vi "AlliGator Phasor Calibration Actions.vi"(0 "AlliGator Q Elements":T6[](array[typedef]), 1 "VI in":refnum<vi>, 2 "Script in":bool, 5 "data value reference":refnum<data-value>, 7 "AlliGator Q Event in":T7=enum."GUI:Idle", 9 "Data":variant, 11 "error in (no error)":errorcluster, 12 "AlliGator Ctrl Refnums":T8) -> (3 "Script out":bool, 4 "Alligator Queue Element 1 (+ 2)":T6[](array[typedef]), 6 "AlliGator IV DVR":refnum<data-value>, 10 "[Notebook Message]":T1[](array[typedef]) {"Message Style"."Font Size" min=6.0 step=1.0}, 15 "error out":errorcluster)   [LabVIEW 2021, in "AlliGator Action Engine.lvlib"]
doc: "Processes AlliGator phasor calibration-related actions."
uses:
  AlliGator Action Engine.lvlib
  Internal Variables/AlliGator Internal Variables v2.ctl
  <vilib>/vision/Image Controls.llb/IMAQ Image.ctl
  Internal Variables/AlliGator Gate Image Set.ctl
  Files/AlliGator FLI Dataset Type.ctl
  Files/AlliGator Data Series Type.ctl
  Dual-Channel Datasets/AlliGator Dataset Channel.ctl
  Settings/AlliGator Gate Arithmetic.ctl
  Source Image/AlliGator Displayed Image.ctl
  Image/Named ROI Description.ctl
  Phasor Graph/AlliGator Decay Metadata v3.ctl
  Decay Analysis/Decay Preprocessing/AlliGator Decay Background Subtraction Info.ctl
  Decay Analysis/Decay Preprocessing/AlliGator Baseline Subtraction Method.ctl
  Graphs/XY Graph/XY Graph Plot Shift Parameters.ctl
  Graphs/XY Graph/XY Graph Plot Shift Method.ctl
  Decay Analysis/Decay Preprocessing/AlliGator Decay Extrapolation Parameters.ctl
  Phasor/Calibration Phasor (m, phi).ctl
  Phasor/Phasor Reference Series.ctl
  Phasor/Phasor Calibration Map v2.ctl
  Phasor/Phasor (g, s).ctl
  Phasor Graph/AlliGator Raw Phasor Plot Data v5.ctl
  Phasor/Phasor Standard Deviation Options.ctl
  Phasor Plot/AlliGator Phasor Multi-Harmonic Data.ctl
  Phasor/Phasor Harmonic Data.ctl
  Decay Fit Parameter Map/AlliGator Decay Fit Options & Parameters v4.ctl
  Fits/IRF(X)PSED/Decay Fit Options v4.ctl
  Fits/Decay Convolution/Decay Model.ctl
  Fits/Residual Type.ctl
  Fits/IRF(X)PSED/Fit Weights Type v2.ctl
  Fits/Non-linear Fitting Method v2.ctl
  Fits/Fit Calculation Method.ctl
  Fits/Non-linear Fitting Algorithm.ctl
  Decay Analysis/Decay Fit/AlliGator Decay Fit Parameter Constraints 2.ctl
  Fits/IRF(X)PSED/Decay Fit Parameters In List.ctl
  Fits/IRF(X)PSED/MLE Baseline Offset Type.ctl
  Decay Analysis/Decay Preprocessing/AlliGator Decay Preprocessing Parameters.ctl
  Fits/IRF(X)PSED/Decay Fit Parameters & Derived Quantities List v2.ctl
  Fits/IRF(X)PSED/Decay Fit Result Constraint.ctl
  Decay Fit Parameter Map/AlliGator Parameter Maps Data.ctl
  AlliGator Q Event.ctl
  GUI/AlliGator Ctrl Refnums.ctl
  GUI/AlliGator Other Ctrl Refnums.ctl
  GUI/AlliGator State Indicator.ctl
  GUI/AlliGator Main Window Tabs.ctl
  GUI/AlliGator Phasor Plot Ctrl Refnums.ctl
  GUI/AlliGator Phasor Graph Ctrl Refnums.ctl
  Phasor/Phasor Calibration Type.ctl
  GUI/AlliGator Dataset Ctrl Refnums.ctl
  GUI/AlliGator Registered Events Ctrl Refnums.ctl
  GUI/AlliGator Image Histogram Control Refnums.ctl
  Histograms/Linear Histogram Options.ctl
  Histograms/Histogram Bin Option.ctl
  Histograms/Histogram Bin Position.ctl
  Decay Fit Parameter Map/AlliGator Decay Fit Map Control Refnums.ctl
  Parameter Map/AlliGator Parameter Map Control Refnums.ctl
  AlliGator Q Element.ctl
  Notebook/Notebook Message Object.ctl
  Rich Text Box/Text Formatting.ctl
  Rich Text Box/Text Colors.ctl
  Rich Text Box/Text Style.ctl
  Rich Text Box/Text Alignment.ctl
  Alligator Elements Order in Action Stack.ctl
  AlliGator State Indicators List.ctl
  Rich Text Box/Text Format List.ctl
  Graphs/XY Graph/XY Graph Mouse Click Event Data.ctl
  Graphs/XY Graph/XY Graph Refnum.ctl
  <vilib>/Utility/miscctls.llb/LVPoint32TypeDef.ctl
  Files/Load-Save File Info.ctl
  Variant/Variant to Data/Variant to I32.vi
  Variant/Variant to Data/Variant to Boolean.vi
  AlliGator Add Single Action to Stack.vi
  Graphs/Get Plot at Mouse Click (XY Graph)/Get Plot at Mouse Click [AAC].vi
  AlliGator Add Action Array to Stack.vi
  Phasor/Phasor.lvlib
  Settings/AlliGator Settings.lvlib
  Phasor Calibration/AlliGator Phasor Calibration.lvlib
  Files/Files.lvlib
  GUI/AlliGator GUI.lvlib
  Graphs/XY Graph/XY Graph Add-Ons.lvlib
  Graphs/Graphs.lvlib
  GUI/GUI.lvlib
  Phasor Graph/AlliGator Phasor Graph.lvlib
  Variant/Variant to Data/Variant to Data.lvlib
  Internal Variables/AlliGator Internal Variables.lvlib
  Sound/Sound.lvlib
  Notebook/Notebook.lvlib
  Source Image/AlliGator Source Image.lvlib
  Decay Fit Parameter Map/AlliGator Decay Fit Parameter Map.lvlib
  Image/Image.lvlib
  Decay Analysis/Decay Preprocessing/AlliGator Decay Preprocessing.lvlib
  Files/AlliGator Files.lvlib
  Phasor Plot/AlliGator Phasor Plot.lvlib
  Fits/Fits.lvlib
  Decay Analysis/Decay Fit/AlliGator Decay Fit.lvlib
  Rich Text Box/Rich Text Box.lvlib
  Dual-Channel Datasets/AlliGator Dual-Channel Datasets.lvlib
  Histograms/Histogram Window.lvlib
  Parameter Map/AlliGator Parameter Map.lvlib
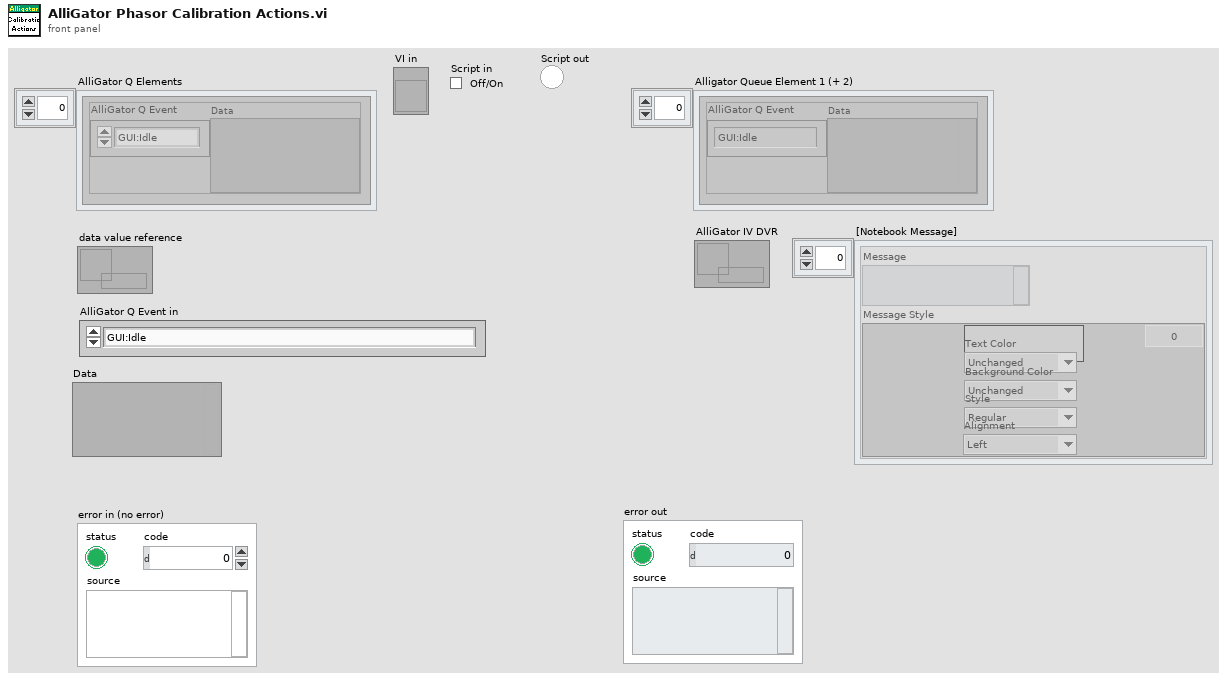
[diagram p1: front panel]
types:
  T1 = typedef "Notebook.lvlib/Notebook Message Object.ctl" = cluster{"Message":string, "Message Style":T2}
  T2 = typedef "Rich Text Box.lvlib/Text Formatting.ctl" = cluster{"Font":string, "Text Color":T3, "Background Color":T3, "Style":T4, "Font Size":dbl, "Alignment":T5}
  T3 = typedef "Rich Text Box.lvlib/Text Colors.ctl" = enum16{"Unchanged", "Black", "Blue", "Cyan", "Maroon", "Gray", "Violet", "Green", "Light Green", "Orange", "Yellow", "Magenta", "Red", "White"}
  T4 = typedef "Rich Text Box.lvlib/Text Style.ctl" = enum16{"Regular", "Bold", "Italic", "Underline", "Strikeout"}
  T5 = typedef "Rich Text Box.lvlib/Text Alignment.ctl" = enum16{"Left", "Right", "Center"}
  T6 = typedef "AlliGator Action Engine.lvlib/AlliGator Q Element.ctl" = cluster{"AlliGator Q Event":T7, "Data":variant}
  T7 = typedef "AlliGator Action Engine.lvlib/AlliGator Q Event.ctl" = enum16{"---- Files ----", "Files:Set Batch Export Files To Save", "Files:Set Dataset Loading & Pre-processing Options", "Files:Check #Frames in Dataset", "Files:Increment Frame Index", "Files:Open Mask Image", "Files:Open White Light Image", "Files:Open Single Dataset", "Files:New Folder of Folders Selected", "Files:Load File (all Types)_Scriptable", "Files:Move Flattened Series to Folders Series", "Files:Select Folder", "Files:Load FLI Dataset", "Files:Load Swiss SPAD 1 Dataset", "Files:Load Swiss SPAD 2 Dataset", "Files:Load .sdt FLI Dataset", "Files:Load .ptu FLI Dataset", "Files:Load .bin FLI Dataset", "Files:Load Single Gate Image Folder", "Files:Load I/m/phi Dataset (deprecated)", "Files:Load Single Image", "Files:Subtract Background File", "Files:Export FLI Dataset", "Files:Load HDF5 FLI Dataset", "Files:Set Destination File Path", "Files:Save Mask Image", "Files:Batch Conversion", "Files:New Folder Selected", "Files:Close FLI Dataset", "Files:Close FLI Dataset Series", "Files:Close White Light Image", "Files:Close Mask Image", "---- FLI Dataset ----", "FLI Dataset:Channel Arithmetic", "FLI Dataset:Export Average Lifetime Map as ASCII", "FLI Dataset:Export User-Defined Quantity Map as ASCII", "FLI Dataset:Python Function FLI Dataset Event", "FLI Dataset:ROI Analysis", "FLI Dataset:Tilted Logistic Square Gated IRF Characteristics Map", "FLI Dataset:Logistic Square Gated IRF Characteristics Map", "FLI Dataset:Square Gated IRF Characteristics Map", "FLI Dataset:Multi-ROI Single-Pixel Phasor Analysis", "FLI Dataset:Multi-ROI Single-Pixel NLSF Analysis", "FLI Dataset:All ROIs IRF Extraction", "FLI Dataset:All ROIs Decay Fit Non-Interactive (Fast + Individual IRF)", "FLI Dataset:All ROIs Phasor Analysis", "FLI Dataset:All ROIs Decay Fit", "FLI Dataset:Fluorescence Decay Statistics", "FLI Dataset:Update Decay Statistics Graph", "FLI Dataset:Get Decay from ROI", "FLI Dataset:All ROIs Average Lifetimes", "FLI Dataset:Save/Load Local IRFs", "FLI Dataset:Clear Local IRFs", "FLI Dataset:Phasor Calibration Maps (# Gates Series) Script", "FLI Dataset:Calibrated Phasor Map Series", "---- FLI Dataset Series ----", "FLI Dataset Series:Sum All Datasets in Series", "FLI Dataset Series:Add Dataset to Accumulated Dataset", "FLI Dataset Series:Display Accumulated Dataset", "FLI Dataset Series:Clear Dataset Series Sum", "FLI Dataset Series:Time-Series Analysis (NLSF)", "FLI Dataset Series:Time-Series Analysis (Phasor)", "---- Image ----", "Image:Update Image Profile Plots", "Image:Image Histogram Cursor Move", "Image:Image Histogram", "Image:Image Contrast", "Image:Set Image Histogram Cursor Move Flag", "Image:Clear Image Overlay", "Image:Use ROI as Search Area", "Image:Set ROI Diameter", "Image:Save Image Data as TIFF", "Image:Save Displayed Image with Overlay", "Image:Save Image Overlay Only", "Image:Save Image as Hot Pixel Mask", "Image:Change Source Image Color Palette", "Image:Copy Image to Clipboard", "Image:Source Image ROI Selection", "Image:Delete All ROIs", "Image:Delete All Unselected ROIs", "Image:Delete ROI", "Image:Merge All ROIs", "Image:Store ROI", "Image:Source Image ROI Storage", "Image:Export ROI Description to Notebook", "Image:Save ROI", "Image:Load ROI", "Image:Paste ROI Definition", "Image:Clear ROI", "Image:Identify ROIs in Mask Image", "Image:Create Complementary ROI", "Image:Create Contour ROI", "Image:Create ROI(s) from Pixels with Peak above Min_Scriptable", "Image:Create ROI(s) from Pixels with Intensity above Min_Scriptable", "Image:Compute ROI Statistics", "Image:Delete ROI(s) based on ROI Characteristics", "Image:Create ROI Grid", "Image:ROI to Individual Pixel ROIs", "Image:Python Function Source Image Event", "Image:Show Phasor Calibration Map ROI Centers", "Image:Convert ROI to Mask Image", "Image:Mouse Move", "Image:Mouse Up", "Image:Set Source Image Mouse Move Flag", "Image:Add Scale Bar Overlay", "Image:Delete Existing ROIs Option", "Image:Overlay ROI Median", "Image:Check Current ROI", "Image:Update True Pixel Value", "---- Decay ----", "Decay:Clear IRF/Reference Plot", "Decay:Add Decay to Graph", "Decay:Smoothen Plot", "Decay:Smoothen Plot Tail", "Decay:Average Selected Plots", "Decay:Extract IRF", "Decay:Optimal IRF Extraction", "Decay:Threshold IRF", "Decay:Fit to Model IRF", "Decay:Fit IRF to Square Gate", "Decay:Fit IRF to Logistic Square Gate", "Decay:Fit IRF to Tilted Logistic Square Gate", "Decay:Create Bounding Cursors Set", "Decay:Export Bounding Cursors Definition to Notebook", "Decay:Denoise Plot", "Decay:Compute Cumulative Function", "Decay:Use as Reference Decay", "Decay:Show Reference Decay/IRF", "Decay:Extrapolate Decay", "Decay:Create Head & Tail Bounding Cursors", "Decay:Store Cursor-defined Head & Tail Fractions", "Decay:Rebin Plot", "Decay:1-Normalize Decay", "Decay:[0-1]-Normalize Plot", "Decay:Straighten Decay", "Decay:Shift Decay", "Decay:Fold Decay", "Decay:Fit Decay", "Decay:Global Fit of Selected Decays", "Decay:Post Global Fit Script", "Decay:Add Global Fit Parameters to Graph", "Decay:Add Decay Parameter(s) to Plot (Graph)", "Decay:Export Decay to Phasor Graph", "Decay:Compute Average Lifetime", "Decay:Plot Convolution", "Decay:Graph Tip Strip Update", "---- Decay Statistics ----", "Decay Statistics:Tip Strip Update", "---- Intensity Time Trace ----", "Intensity Time Trace:Use File Timestamp", "Intensity Time Trace:Load Intensity Corrections File", "Intensity Time Trace:Clear Intensity Corrections File", "Intensity Time Trace:Tip Strip Update", "---- Phasor Plot ----", "Phasor Plot:Build Phasor Plot", "Phasor Plot:Change Phasor Plot Color Palette", "Phasor Plot:Adjust Phasor Plot Display Range", "Phasor Plot:Highlight Image ROI in Phasor Plot", "Phasor Plot:Save Phasor Plot Image with Overlay", "Phasor Plot:Export Complex Phasor Map", "Phasor Plot:Export Phasor Ratio Map", "Phasor Plot:Export Average Lifetime Map", "Phasor Plot:Compute Phase Lifetime Histogram", "Phasor Plot:Compute Phasor Ratio Histogram", "Phasor Plot:Compute Phase Lifetime vs Intensity Scatter Plot", "Phasor Plot:Weber 2-Component Decomposition", "Phasor Plot:Update Phasor Color Map Vertices", "Phasor Plot:Clear Phasor Overlay", "Phasor Plot:Use Segment Extremities as References", "Phasor Plot:Use UC/Segment Intersections as References", "Phasor Plot:Use UC/Principal Axis Intersections as References", "Phasor Plot:Use UC/Linear Fit Intersections as References", "Phasor Plot:Update Phasor Plot Reference", "Phasor Plot:Show Local Phasor Info in Phasor Plot", "Phasor Plot:Update Phasor Plot State", "Phasor Plot:Phasor Plot ROI Storage", "Phasor Plot:Phasor Plot ROI Selection", "Phasor Plot:Python Function Phasor Plot Event", "Phasor Plot:Overlay Phasor ROI, Ratio or Map in Source Image", "Phasor Plot:Compute Decay of Selected Phasors", "Phasor Plot:Phasor at Image Pixel", "Phasor Plot:Mouse Move", "Phasor Plot:Mouse Up", "Phasor Plot:Display Range Mouse Move", "Phasor Plot:Set Mouse Move Flag", "Phasor Plot:Update True Phasor Plot Value", "---- Phasor Graph ----", "Phasor Graph:Get Phasor Value", "Phasor Graph:Create New Phasor Plot Dialog", "Phasor Graph:Update Last Phasor Value", "Phasor Graph:Update Phasor (m, phi)", "Phasor Graph:Remove Single Phasor from Plot", "Phasor Graph:Add Single Phasor to Plot", "Phasor Graph:Remove Phasor Plot", "Phasor Graph:Remove Selected Phasor Plots", "Phasor Graph:Clear Phasor Data", "Phasor Graph:Clear Phasor Graph", "Phasor Graph:Cursor Move", "Phasor Graph:Draw Cursor Connecting Line", "Phasor Graph:Clear Cursor Connecting Line", "Phasor Graph:Find UC Intersection", "Phasor Graph:Use UC/Cursor-Defined Line Intersections", "Phasor Graph:Use Selected Plots Fitted Line/UC Intersections", "Phasor Graph:Use Selected Plots Principal Axis/UC Intersections", "Phasor Graph:Show Single Phasor", "Phasor Graph:Save Single Phasor Plot", "Phasor Graph:Save All Phasor Plots", "Phasor Graph:Load Phasor Plot(s)", "Phasor Graph:Phasor Multiplication", "Phasor Graph:Compute Average Phasor", "Phasor Graph:Compute Multiple Average Phasors (Selected Plots)", "Phasor Graph:Export Single Phasor Plot Phase Lifetimes", "Phasor Graph:Parameter 2 vs Parameter 1 Scatter Plot", "Phasor Graph:Use Cursor n Location", "Phasor Graph:Set Reference n to Current Phase Lifetime Value", "Phasor Graph:Set Reference n to Lifetime Value", "Phasor Graph:Set Cursor n Location", "Phasor Graph:Save Phasor Graph Image", "Phasor Graph:Update SEPL Plot", "Phasor Graph:Export Single Phasor Plot Data", "Phasor Graph:Export Selected Phasor Plots Data", "Phasor Graph:Python Function Phasor Graph Event", "Phasor Graph:Tip Strip Update", "---- Calibration ----", "Calibration:Set Calibration Type", "Calibration:Load/Save Phasor Calibration", "Calibration:Load/Save Phasor Calibration Series", "Calibration:Load/Save Phasor Calibration Map", "Calibration:Use as Calibration", "Calibration:Compute Optimal Calibration from Phasor References", "Calibration:Clear Phasor Calibration", "Calibration:Single Phasor Calibration Information", "Calibration:Use as Calibration Series", "Calibration:Use as Calibration Map", "Calibration:Clear Calibration Series", "Calibration:Phasor Calibration Series Information", "Calibration:Clear Calibration Map", "Calibration:Phasor Calibration Map Information", "Calibration:Apply Phasor Calibration", "Calibration:Update Single Plot Calibration", "Calibration:Update Multiple Plots Calibration", "Calibration:Clear Single Plot Calibration", "Calibration:Clear All Plots Calibrations", "Calibration:Clear Plot(s) Calibration(s)?", "---- Phasor Ratio ----", "Phasor Ratio:Clear Reference n", "Phasor Ratio:Toggle Selected Plot(s)  Lock to Reference 1", "Phasor Ratio:Use as Reference n", "Phasor Ratio:Send Reference n to Notebook", "Phasor Ratio:Toggle Selected Plot(s)  Lock to Reference 2", "Phasor Ratio:Compute Phasor Ratio at Mouse Location", "Phasor Ratio:Compute Phasor Plot's Average Phasor Ratio", "Phasor Ratio:Compute Time-Series Phasor Ratios", "Phasor Ratio:Fit Line to Phasor Ratio Plot", "Phasor Ratio:Save References", "Phasor Ratio:Load References", "Phasor Ratio:Update Phasor Reference 1", "Phasor Ratio:Update Phasor Reference 2", "Phasor Ratio:Move Cursor n to Reference n", "Phasor Ratio:Use as Phasor Reference 1 Lifetime", "Phasor Ratio:Use as Phasor Reference 2 Lifetime", "Phasor Ratio:Export Phasor Ratio Map as ASCII", "Phasor Ratio:Tip Strip Update", "---- Lifetime & Other Parameters Graph ----", "Lifetime:Compute Sliced Mean, SDV and CV Plots", "Lifetime:Plot Decay Shifts", "Lifetime:Plot Histogram", "---- Decay Fit Parameter Map ----", "Decay Fit Parameter Map:Export ROI NLSF Data as ASCII", "Decay Fit Parameter Map:Set Decay Fit Parameter Map Selection", "Decay Fit Parameter Map:Build Decay Fit Parameter Map", "Decay Fit Parameter Map:Change Decay Fit Parameter Map Color Palette", "Decay Fit Parameter Map:Export Decay Fit Parameter Map Data as ASCII", "Decay Fit Parameter Map:Export All Decay Fit Parameter Maps Data as ASCII", "Decay Fit Parameter Map:Selected Parameter Scatterplot", "Decay Fit Parameter Map:Parameter 2 vs Parameter 1 Scatterplot", "Decay Fit Parameter Map:Save Decay Fit Parameter Map Image", "Decay Fit Parameter Map:Save-Load IRFs & Fit Data", "Decay Fit Parameter Map:Update Local Decay Plots", "Decay Fit Parameter Map:Python Function Decay Fit Parameters Map Event", "Decay Fit Parameter Map:Overlay Decay Fit Parameter Map in Source Image", "Decay Fit Parameter Map:Selected Parameter vs Intensity Scatterplot", "Decay Fit Parameter Map:Mouse Up", "Decay Fit Parameter Map:Mouse Move", "Decay Fit Parameter Map:Display Range Mouse Move", "Decay Fit Parameter Map:Change Map Resolution", "Decay Fit Parameter Map:Variance Significance Maps", "Decay Fit Parameter Map:Fit Result Constraints Window", "---- Parameter Map ----", "Parameter Map:Export ROI Parameters Data as ASCII", "Parameter Map:Add Parameter Map Set", "Parameter Map:Delete Parameter Map Set", "Parameter Map:Update Parameter List", "Parameter Map:Build Parameter Map", "Parameter Map:Change Parameter Map Color Palette", "Parameter Map:Export Parameter Map Data as ASCII", "Parameter Map:Export All Parameter Maps Data as ASCII", "Parameter Map:Selected Parameter Scatterplot", "Parameter Map:Parameter 2 vs Parameter 1 Scatterplot", "Parameter Map:Selected Parameter vs Intensity Scatterplot", "Parameter Map:Save Parameter Map Image", "Parameter Map:Save-Load IRFs & Parameter Maps (TODO)", "Parameter Map:Set Parameter Map Selection", "Parameter Map:Python Function Parameter Map Event", "Parameter Map:Overlay Parameter Map in Source Image", "Parameter Map:Update Local Decay Plots", "Parameter Map:Mouse Up", "Parameter Map:Mouse Move", "Parameter Map:Display Range Mouse Move", "---- Generic Graph ----", "Generic Graph:Generic XY Graph Event", "Generic Graph:Python Function XY Graph Event", "Generic Graph:New Plot", "Generic Graph:Save Plot", "Generic Graph:XY Plot Histogram", "Generic Graph:Set XY Graph Plot Name", "Generic Graph:Set Last Cursor Style", "Generic Graph:Tip Strip Update", "---- GUI ----", "GUI:Start Script", "GUI:Type of Displayed Image Changed", "GUI:Gate Image Slide Changed", "GUI:Show Busy Icon", "GUI:Show Busy Icon & Abort Button", "GUI:Hide Busy Icon", "GUI:Hide Busy Icon & Abort Button", "GUI:Abort", "GUI:End Script", "GUI:Start Timing", "GUI:End Timing", "GUI:Set State Indicator", "GUI:Send Parameters JSON Strings to Clipboard", "GUI:Set Gate Step", "GUI:Idle", "GUI:Initialization", "GUI:Quit", "GUI:Increment Dataset Index", "GUI:Set Dataset Index to -1", "GUI:Time Series Slider Moved", "GUI:Time Series Slider Changed", "GUI:Toggle Playback or Loop", "GUI:Playback Script", "GUI:Set Phasor Frequency", "GUI:Open Window", "GUI:Start Test Script", "GUI:End Test Script", "GUI:Set Verbose Mode", "GUI:Set Verbose Settings Mode", "DEBUG"}
  T8 = typedef "AlliGator GUI.lvlib/AlliGator Ctrl Refnums.ctl" = cluster{"Other AlliGator Ctrl Refnums":T9, "Phasor Plot Ctrl Refnums":T10, "Phasor Graph Ctrl Refnums":T11, "Dataset Control Refnums":T12, "Registered Events Ctrl Refnums":T13, "Image Histogram Ctrl Refnums":T14, "Decay Fit Map Ctrl Refnums":T15, "Parameter Map Ctrl Refnums":T16}
  T9 = typedef "AlliGator GUI.lvlib/AlliGator Other Ctrl Refnums.ctl" = cluster{"State Indicators":refnum<vi>, " Progress Bar":refnum<vi>, "Decay Graph Active":refnum<vi>, "Decay Statistics Bin":refnum<vi>, "Time Step":refnum<vi>, "Use File Timestamp":refnum<vi>, "Tab Control":refnum<vi>, "CPU":refnum<vi>, "Abort Fit":refnum<vi>, "Dataset File/Folder Path":refnum<vi>, "Abort ROI Creation":refnum<vi>, "Event LED":refnum<vi>, "Dataset File/Folder Path 2":refnum<vi>, "Dataset File/Folder Path 3":refnum<vi>, "Dataset File/Folder Path 4":refnum<vi>, "Dataset File/Folder Path 5":refnum<vi>, "Dataset File/Folder Path 6":refnum<vi>, "Dataset File/Folder Path 7":refnum<vi>, "Dataset File/Folder Path 8":refnum<vi>, "Dataset File/Folder Path 9":refnum<vi>, "Dataset File/Folder Path 10":refnum<vi>, "Dataset File/Folder Path 11":refnum<vi>}
  T10 = typedef "AlliGator GUI.lvlib/AlliGator Phasor Plot Ctrl Refnums.ctl" = cluster{"Phasor Ratio":refnum<vi>, "Modulus Lifetime":refnum<vi>, "Phasor at cursor (m, phi)":refnum<vi>, "Phase Lifetime":refnum<vi>, "Phasor at cursor (g, s)":refnum<vi>, "Phasor Plor Average Lifetime":refnum<vi>, "Phasor Plot Active":refnum<vi>, "Save Phasor Plot":refnum<vi>, "Image Overlay Color":refnum<vi>, "Phasor Plot Color Scale":refnum<vi>, "Reference 1 Button":refnum<vi>, "Reference 2 Button":refnum<vi>, "True Phasor Plot Value":refnum<vi>}
  T11 = typedef "AlliGator GUI.lvlib/AlliGator Phasor Graph Ctrl Refnums.ctl" = cluster{"Phasor Ratio":refnum<vi>, "Modulus Lifetime":refnum<vi>, "Phasor at cursor (m, phi)":refnum<vi>, "Phase Lifetime":refnum<vi>, "Phasor at cursor (g, s)":refnum<vi>, "Phasor Graph Average Lifetime":refnum<vi>, "Phasor Graph Active":refnum<vi>, "Save Phasor Graph":refnum<vi>, "Phasor Frame Slide":refnum<vi>, "Single Step Phasor":refnum<vi>, "Calibration Type":refnum<vi>, "Show Line":refnum<vi>, "Phase Lifetime 1":refnum<vi>, "Phase Lifetime 2":refnum<vi>, "Phasor Graph Frequency":refnum<vi>, "Phasor Reference 1 Control":refnum<vi>, "Phasor Reference 2 Control":refnum<vi>, "Calibration Lifetime":refnum<vi>, "Phase Lifetime SDV":refnum<vi>, "Average Lifetime SDV":refnum<vi>, "Phasor Ratio SDV":refnum<vi>, "Modulus Lifetime SDV":refnum<vi>}
  T12 = typedef "AlliGator GUI.lvlib/AlliGator Dataset Ctrl Refnums.ctl" = cluster{"Current Data":refnum<vi>, "Gate Image Slide":refnum<vi>, "Time Point Slide":refnum<vi>, "Current Time Stamp":refnum<vi>, "Save Image":refnum<vi>, "Displayed Image":refnum<vi>, "Overlay Mode":refnum<vi>, "Phasor Overlay Color":refnum<vi>, "Image Color Scale":refnum<vi>, "Use ROI as Search Area":refnum<vi>, "Source Image ROI Color":refnum<vi>, "True Pixel Value":refnum<vi>}
  T13 = typedef "AlliGator GUI.lvlib/AlliGator Registered Events Ctrl Refnums.ctl" = cluster{"Time Point Slider":refnum<vi>, "Phasor Plot Display Range":refnum<vi>, "Decay Graph":refnum<vi>, "Decay Statistics Graph":refnum<vi>, "Intensity Time Trace":refnum<vi>, "Phasor Graph":refnum<vi>, "Phasor Ratio Graph":refnum<vi>, "Lifetime Graph":refnum<vi>, "Phasor Plot Display":refnum<vi>, "Source Image Display":refnum<vi>, "Decay Fit Parameter Map Display Range":refnum<vi>, "Decay Fit Parameter Map Display":refnum<vi>, "Parameter Map Display Range":refnum<vi>, "Parameter Map Display":refnum<vi>, "Phasor Plot Display Range":refnum<vi>}
  T14 = typedef "AlliGator GUI.lvlib/AlliGator Image Histogram Control Refnums.ctl" = cluster{"Image Histogram":refnum<vi>, "Image Histogram Options":refnum<vi>, "Image Histogram Active":refnum<vi>, "Image Histogram Upper Percentile":refnum<vi>, "Image Histogram Lower Percentile":refnum<vi>, "Auto-Adjust Contrast":refnum<vi>}
  T15 = typedef "AlliGator Decay Fit Parameter Map.lvlib/AlliGator Decay Fit Map Control Refnums.ctl" = cluster{"Decay Fit Parameter Map Color Scale":refnum<vi>, "Decay Fit Parameter":refnum<vi>, "Max Parameter":refnum<vi>, "Min Parameter":refnum<vi>, "Decay Fit Parameter Map Display":refnum<vi>, "Decay Fit Parameter Map Display Range":refnum<vi>, "Decay Parameter Map X":refnum<vi>, "Decay Parameter Map Y":refnum<vi>, "Decay Parameter Map Value":refnum<vi>}
  T16 = typedef "AlliGator Parameter Map.lvlib/AlliGator Parameter Map Control Refnums.ctl" = cluster{"Parameter Map Color Scale":refnum<vi>, "Map Parameter":refnum<vi>, "Max Parameter":refnum<vi>, "Min Parameter":refnum<vi>, "Parameter Map Display":refnum<vi>, "Parameter Map Display Range":refnum<vi>, "Parameter Map Set":refnum<vi>, "Parameter Map X":refnum<vi>, "Parameter Map Y":refnum<vi>, "Parameter Map Value":refnum<vi>}
  T17 = typedef "AlliGator Action Engine.lvlib/Alligator Elements Order in Action Stack.ctl" = enum16{"Enqueue 2 AFTER 1", "Enqueue 2 BEFORE 1"}
  T18 = typedef "AlliGator Action Engine.lvlib/AlliGator State Indicators List.ctl" = enum16{"Phasor Calibration Defined", "Phasor Calibration Series Defined", "Phasor Calibration Map Defined", "Phasor Reference 1 Defined", "Phasor Reference 2 Defined", "Lifetime Reference 1 Defined", "Lifetime Reference 2 Defined", "Phasor Calibration Used", "Phasor Calibration Series Used", "Phasor Calibration Map Used", "Dataset Update Needed", "Phasor Plot Update Needed", "Reference/IRF Defined", "Individual IRFs Defined"}
  T19 = typedef "Phasor.lvlib/Phasor Calibration Map v2.ctl" = cluster{"Phasor Frequency":dbl[unit], "Calibration Lifetime":dbl[unit], "ROI Centers":cluster{"X":i32, "Y":i32}[], "ROI Descriptors":T20[], "Map Resolution X":i32, "Map Resolution Y":i32, "z Array":cdb[]}
  T20 = typedef "ROI Descriptor" = cluster{"Global Rectangle":i32[], "Contours":cluster{"ID":enum32{"External", "Internal"}, "Type":u32, "Coordinates":i32[]}[]}
  T21 = typedef "Notebook.lvlib/Text Format List.ctl" = enum16{"Message", "Result", "Error", "Setting", "Verbose", "Warning"}
  T22 = typedef "Phasor.lvlib/Phasor Reference Series.ctl" = cluster{"m Array":dbl[], "phi Array":dbl[], "Phasor Frequency":dbl[unit], "Calibration Lifetime":dbl[unit]}
  T23 = typedef "Phasor.lvlib/Calibration Phasor (m, phi).ctl" = cluster{"m":dbl, "phi":dbl, "Phasor Frequency":dbl[unit], "Reference Lifetime":dbl[unit]}
  T24 = typedef "XY Graph Add-Ons.lvlib/XY Graph Mouse Click Event Data.ctl" = cluster{"Multiplot XY Graph":T25, "Mouse Coordinates":T26}
  T25 = typedef "XY Graph Add-Ons.lvlib/XY Graph Refnum.ctl" = refnum<vi>
  T26 = typedef "LVPoint32TypeDef.ctl" = cluster{"Horizontal":i32, "Vertical":i32}
  T27 = typedef "Files.lvlib/Load-Save File Info.ctl" = cluster{"Load/Save":bool, "File Path":path}
  T28 = typedef "Phasor.lvlib/Phasor Calibration Type.ctl" = enum16{"None", "Single Phasor", "Phasor Series", "Phasor Map"}
  T29 = typedef "Phasor.lvlib/Phasor (g, s).ctl" = cluster{"g":dbl, "s":dbl}
  T30 = typedef "AlliGator Internal Variables.lvlib/AlliGator Internal Variables v2.ctl" = cluster{"----------------------------- Images -----------------------------":u8, "Displayed Image":T31, "White Light Image":T31, "Mask Image":T31, "ROI Mask Image":T31, "Current Dataset Images 1":T32, "Background Dataset Images 1":T32, "Current Dataset Images 2":T32, "Background Dataset Images 2":T32, "Current Dataset Arithmetic Images":T32, "Accumulated Dataset Images 1":T32, "Accumulated Dataset Images 2":T32, "Accumulated Dataset Arithmetic Images":T32, "----------------------------- File Paths -----------------------------":u8, "Phasor Plot Image":T31, "Decay Fit Parameter Map Image":T31, "Parameter Map Image":T31, "Single Data Point Path":path, "White Light Image Path":path, "Mask Image Path":path, "Time-Series Folder":path, "[Time-Series Paths]":path[], "----------------------------- FLI Dataset -----------------------------":u8, "Current Dataset":i32, "Single Dataset Type":T33, "Current Folder":string, "AlliGator Data Series Type":T34, "# Datasets":i32, "Dual-Channel Dataset":bool, "Selected Channel Name":string, "Dataset Channel":T35, "Channel Arithmetic":T36, "Dual-Channel Background Dataset":bool, "Background Channel":T35, "Dual-Channel Accumulated Dataset":bool, "Start Time":dbl, "[Time-Series Timestamps]":dbl[], "[Intensity Corrections]":dbl[], "Time Series Script":bool, "Type of Displayed Image":T37, "Gate Image Slide":u16, "# Gates":i32, "ROIs":T38[], "----------------------------- Decays -----------------------------":u8, "ROI Decay":cluster{"t Array":dbl[], "I Array":dbl[]}, "Valid Decay":bool, "Decay  Metadata":T39, "Reference Decay Plot Name":string, "Reference Decay":cluster{"t Array":dbl[], "I Array":dbl[]}, "Decay Shift Plot":cluster{"Time Stamps":dbl[], "Decay Shifts":dbl[]}, "[Decays Max Values]":sgl[], "[Decays Min Values]":sgl[], "----------------------------- Calibration -----------------------------":u8, "Calibration Phasor":T23, "Calibration Phasor Series":T22, "Phasor Calibration Map":T19, "Calibration Map MD5 Digest":string, "----------------------------- Phasor Graph -----------------------------":u8, "Last Raw Phasor":T29, "Last Calibrated Phasor":T29, "Last Calibrated Phasor SDV":T29, "Phasor Graph:Phasor Plot":cluster{"g Array":dbl[], "s Array":dbl[]}, "Phasor Graph:Phasor SDV Plot":cluster{"g Array":dbl[], "s Array":dbl[]}, "[Phasor Graph:Raw Phasor Plots]":T45[], "Phasor Plot locked to Ref 1":i32, "[Phasor Plot(s) locked to Ref 1]":i32[], "[Phasor Plot(s) locked to Ref 2]":i32[], "[Pixel Phasors]":T29[], "----------------------------- Phasor Plot -----------------------------":u8, "[[Sum Image]]":dbl[][], "[[CSG Phasors]]":csg[][], "[[Valid Pixel?]]":bool[][], "[[Phasor Ratios]]":dbl[][], "[[Average Lifetimes]]":dbl[][], "Amplitude Weighted Average Lifetime":bool, "I/m/phi Dataset":cluster{"I/m/phi Dataset?":bool, "Base Frequency":dbl[unit], "Harmonic Orders":u8[]}, "Multi Phasor Plot Data":T47, "----------------------------- Decay Fit Parameter Map -----------------------------":u8, "Decay Fit Options & Parameters":T49, "Fit Options: Decay Preprocessing Parameters":T60, "Fit Options: Reference Decay":cluster{"t Array":dbl[], "I Array":dbl[]}, "Is Full Image Parameters Map":bool, "Is Single-Pixels Parameters Map":bool, "NLSF Parameters Map X Resolution":i32, "NLSF Parameters Map Y Resolution":i32, "[Single Decay Fit Parameters]":dbl[], "Fit Model":T51, "[[Multiple Decays Fit Parameters]]":dbl[][], "[[Multiple Decays Fit Parameter SDVs]]":dbl[][], "[[IRFs]]":dbl[][], "[ROI Descriptors]":T20[], "IRF Array Time Axis":dbl[], "Decay Array Time Axis":dbl[], "[Decay Fit Parameter Names]":T61[], "[Decay Sum]":dbl[], "Array of Decay Fit Result Constraints":T62[], "Selected ROIs Array":bool[], "----------------------------- Parameter Maps -----------------------------":u8, "[Map Set Names]":string[], "[Parameter Maps]":T63[], "[[User-defined Quantities]]":dbl[][], "User-defined Quantity":string}
  T31 = typedef "IMAQ Image.ctl" = refnum<image>
  T32 = typedef "AlliGator Internal Variables.lvlib/AlliGator Gate Image Set.ctl" = cluster{"SGL Gate Images":T31[], "SGL Sum Image":T31, "SGL Max Image":T31, "SGL Min Image":T31}
  T33 = typedef "AlliGator Files.lvlib/AlliGator FLI Dataset Type.ctl" = enum16{"HDF5 FLI Dataset", "Gate Image Folder", ".sdt FLI Dataset (Becker & Hickl)", ".ptu FLI Dataset (PicoQuant)", "SS1 FLI Dataset", "SS2 FLI Dataset", "I/m/phi Dataset", ".bin FLI Dataset (PicoQuant Binned)", ".bin FLI Dataset (Piccolo Binned)", ".mat FLI Dataset"}
  T34 = typedef "AlliGator Files.lvlib/AlliGator Data Series Type.ctl" = enum16{"Not a Supported Series", "Gate Images Folder Series", "SwissSPAD 2 Dataset Series", "B&H FLI Dataset Series", "PicoQuant PTU FLI Dataset Series", "PicoQuant BIN FLI Dataset Series", "Piccolo hist BIN FLI Dataset Series", "HDF5 FLI Dataset Series"}
  T35 = typedef "AlliGator Dual-Channel Datasets.lvlib/AlliGator Dataset Channel.ctl" = enum16{"G2", "INT"}
  T36 = typedef "AlliGator Settings.lvlib/AlliGator Gate Arithmetic.ctl" = enum16{"None", "INT-G2", "G2/INT*<INT>", "(1 - G2/INT)*<INT>"}
  T37 = typedef "AlliGator Source Image.lvlib/AlliGator Displayed Image.ctl" = enum16{"Single Gate", "Sum of All Gates", "Max of All Gates", "Min of All Gates", "-", "White Ligth Image", "Mask Image"}
  T38 = typedef "Image.lvlib/Named ROI Description.ctl" = cluster{"ROI Descriptor":T20, "ROI Name":string, "Overlay Color":u32}
  T39 = typedef "AlliGator Phasor Graph.lvlib/AlliGator Decay Metadata v3.ctl" = cluster{"ROI Descriptor":T20, "ROI Center":cluster{"X":i32, "Y":i32}, "Decay Background Subtraction Info":T40, "Decay Reverted":bool, "Decay Smoothened":bool, "Decay Straightened":bool, "Fitted Tau (Decay Straightening)":dbl, "Decay Shift Parameters":T42, "Decay Shifted":bool, "Decay Extrapolated":bool, "Decay Extrapolation Parameters":T44, "Decay Normalized":bool, "Fold Decay":bool, "# Folds":u32}
  T40 = typedef "AlliGator Decay Preprocessing.lvlib/AlliGator Decay Background Subtraction Info.ctl" = cluster{"Laser Period":dbl[unit], "Gate Duration":dbl[unit], "Baseline Subtraction Method":T41, "Background Definition Range":cluster{"Min Gate":dbl[unit], "Max Gate":dbl[unit]}, "Total Intensity w/o Bkgd Subtraction":dbl, "Bkgd-subtracted Intensity (exp)":dbl, "# Data Points":i32, "Background/Gate":dbl, "Fitted Lifetime":dbl[unit], "Bkgd-subtracted Intensity (theo)":dbl}
  T41 = typedef "AlliGator Decay Preprocessing.lvlib/AlliGator Baseline Subtraction Method.ctl" = enum16{"Mean", "Min", "Square Gated Single-Exponential", "File", "Constant"}
  T42 = typedef "XY Graph Add-Ons.lvlib/XY Graph Plot Shift Parameters.ctl" = cluster{"Type":T43, "Shift":dbl[unit], "Threshold":dbl, "Rotate":bool}
  T43 = typedef "XY Graph Add-Ons.lvlib/XY Graph Plot Shift Method.ctl" = enum16{"Default", "CFD", "Threshold", "Cross-Correlation"}
  T44 = typedef "AlliGator Decay Preprocessing.lvlib/AlliGator Decay Extrapolation Parameters.ctl" = cluster{"Additional Points":u32, "Head Fraction":dbl, "Fitted Tau":dbl, "Use Periodicity":bool, "Use Cursors":bool, "Tail Fraction":dbl}
  T45 = typedef "AlliGator Phasor Graph.lvlib/AlliGator Raw Phasor Plot Data v5.ctl" = cluster{"Phasor Plot Name":string, "Raw Phasor Plot":T29[], "Phasor Frequency":dbl[unit], "[Decay Metadata]":T39[], "Raw Phasor Plot SDV":T29[], "Phasor SDV Options":T46, "[Calibration Phasor]":T23[], "Intensity Array":dbl[]}
  T46 = typedef "Phasor.lvlib/Phasor Standard Deviation Options.ctl" = cluster{"Compute Estimated SDV":bool, "# Replicas":u32, "Use Estimated Average Phasor":bool}
  T47 = typedef "AlliGator Phasor Plot.lvlib/AlliGator Phasor Multi-Harmonic Data.ctl" = cluster{"Base Frequency":dbl[unit], "# Harmonics":u8, "Harmonic Orders":u8[], "Phasor Plot Settings Checksum":u64, "Phasor Harmonic Data Array":T48[]}
  T48 = typedef "Phasor.lvlib/Phasor Harmonic Data.ctl" = cluster{"Phasor Harmonic Name":string, "Phasor Plot Settings Checksum":u64, "Phasor Frequency":dbl[unit], "Base Frequency":dbl[unit], "Harmonic Order":u8, "Phasor Plot Parameters":string, "Phasor Array [[CSG]]":csg[][], "Dataset File Path":path}
  T49 = typedef "AlliGator Decay Fit Parameter Map.lvlib/AlliGator Decay Fit Options & Parameters v4.ctl" = cluster{"SYNC Period":dbl[unit], "Fit Options":T50, "Fit Parameter Constraints":T57[], "MLE Baseline Offset":dbl, "MLE Baseline Offset Type":T59}
  T50 = typedef "Fits.lvlib/Decay Fit Options v4.ctl" = cluster{"Show Fit Residuals":bool, "Fit Model":T51, "Residual Type":T52, "Max Decay Percentile":dbl, "Min Decay Percentile":dbl, "Show Full Decay":bool, "Weights":T53, "Fitting Method":T54, "Compute Parameter Uncertainties":bool, "Periodic Boundaries":bool, "Model Calculation":T55, "Period":dbl[unit], "Termination Criteria":cluster{"Max Iterations":i32, "Max Function Calls":i32, "Max Time":dbl[unit], "Function Tolerance":dbl, "Parameter Tolerance":dbl, "Gradient Tolerance":dbl, "Min Lambda":dbl, "Max Lambda":dbl, "Initial Tick Count":u32}, "Offset Resolution":dbl[unit], "Use Local IRF":bool, "Fitting Algorithm":T56, "Show Confidence Interval ":bool, "Confidence Level":dbl}
  T51 = typedef "Fits.lvlib/Decay Model.ctl" = enum16{"1-Exponential", "2-Exponentials"}
  T52 = typedef "Fits.lvlib/Residual Type.ctl" = enum16{"Standard", "Normalized", "Reduced"}
  T53 = typedef "Fits.lvlib/Fit Weights Type v2.ctl" = enum16{"Unweighted", "1/Variance (Neyman)", "1/Variance (Pearson)", "Best of All"}
  T54 = typedef "Fits.lvlib/Non-linear Fitting Method v2.ctl" = enum16{"Least Square", "Least Absolute Residual", "Bisquare", "MLE", "-", "Best of All"}
  T55 = typedef "Fits.lvlib/Fit Calculation Method.ctl" = enum16{"Simulation", "Convolution", "Integration"}
  T56 = typedef "Fits.lvlib/Non-linear Fitting Algorithm.ctl" = enum16{"Levenberg-Marquardt", "Trust-Region Dogleg"}
  T57 = typedef "AlliGator Decay Fit.lvlib/AlliGator Decay Fit Parameter Constraints 2.ctl" = cluster{"Fit Parameter":T58, "Min Value":dbl, "Max Value":dbl, "Global":bool, "Used":bool}
  T58 = typedef "Fits.lvlib/Decay Fit Parameters In List.ctl" = enum16{"Offset", "Baseline", "A_1", "tau_1", "A_2", "tau_2"}
  T59 = typedef "Fits.lvlib/MLE Baseline Offset Type.ctl" = enum32{"Absolute", "Percentage"}
  T60 = typedef "AlliGator Decay Preprocessing.lvlib/AlliGator Decay Preprocessing Parameters.ctl" = cluster{"Background Subtraction":bool, "Straighten Decay":bool, "Reverse Gates":bool, "1-Normalized Decay":bool, "Smoothen Decay":bool, "Smoothing Parameter":dbl, "Shift Decay":bool, "Decay Shift Parameters":T42, "Extrapolate Decay":bool, "Additional Points":u32, "Head Fraction":dbl, "Pixel-Normalize Decay":bool, "Use Periodicity":bool, "Use Cursors":bool, "Tail Fraction":dbl, "Use Decay Pre-Processing":bool, "Fold Decay":bool, "# Folds":u32, "[0-1]-Normalized Decay":bool}
  T61 = typedef "Fits.lvlib/Decay Fit Parameters & Derived Quantities List v2.ctl" = enum16{"Offset", "Baseline", "A_1", "tau_1", "A_2", "tau_2", "<tau>_a", "f1_a", "f2_a", "<tau>_i", "f1_i", "f2_i", "-", "R^2", "Chi^2"}
  T62 = typedef "Fits.lvlib/Decay Fit Result Constraint.ctl" = cluster{"Fit Parameter":enum16{"Offset", "Baseline", "A_1", "tau_1", "A_2", "tau_2", "<tau>_a", "f1_a", "f2_a", "<tau>_i", "f1_i", "f2_i", "-", "R^2", "Chi^2", "Max Relative Residual", "<Residual ACF>", "Residual ACF SDV", "tau_2/tau_1"}, "Min Value":dbl, "Max Value":dbl, "Use Constraint":bool}
  T63 = typedef "AlliGator Decay Fit Parameter Map.lvlib/AlliGator Parameter Maps Data.ctl" = cluster{"Map Set Name":string, "[Parameter Names]":string[], "[[Parameters]]":dbl[][], "[[Parameter SDVs]]":dbl[][], "Decay Array Time Axis":dbl[], "[[IRFs]]":dbl[][], "IRF Array Time Axis":dbl[], "X Resolution":i32, "Y Resolution":i32, "Intensity Array":dbl[]}
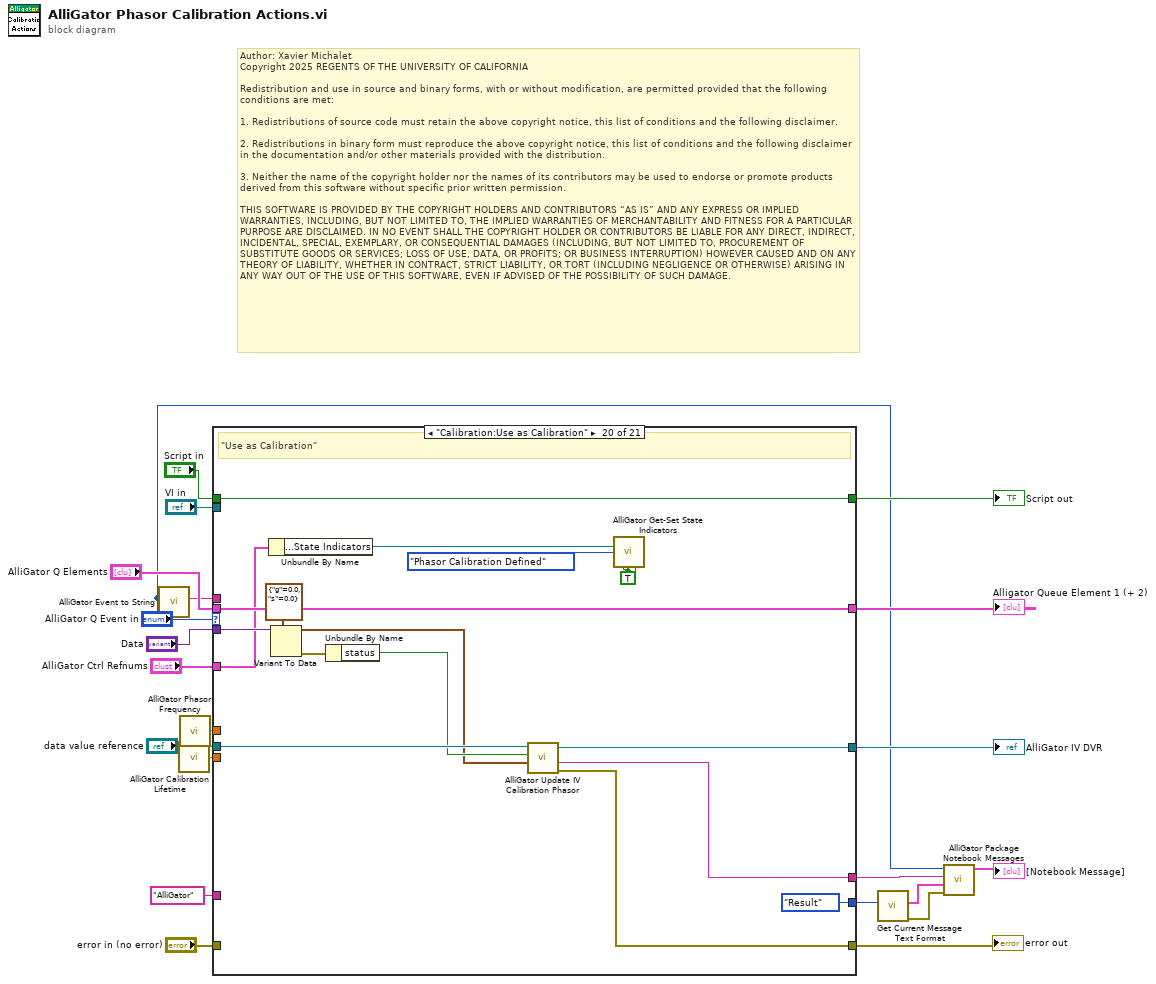
[diagram p0: block diagram]
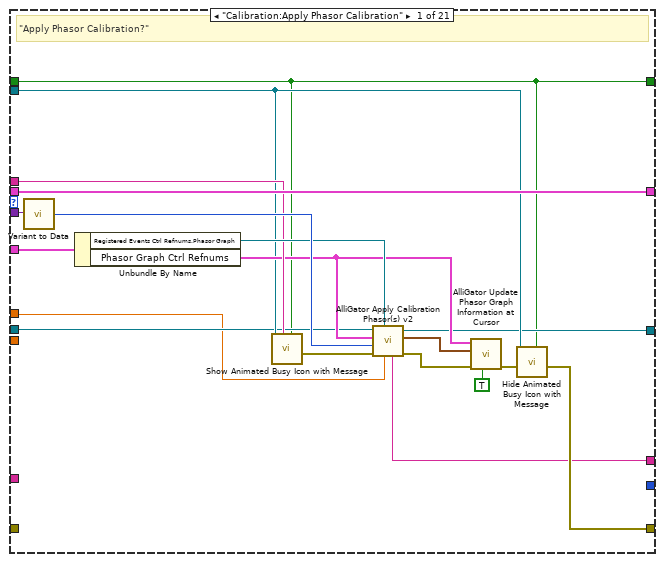
[diagram p2: hidden frame]
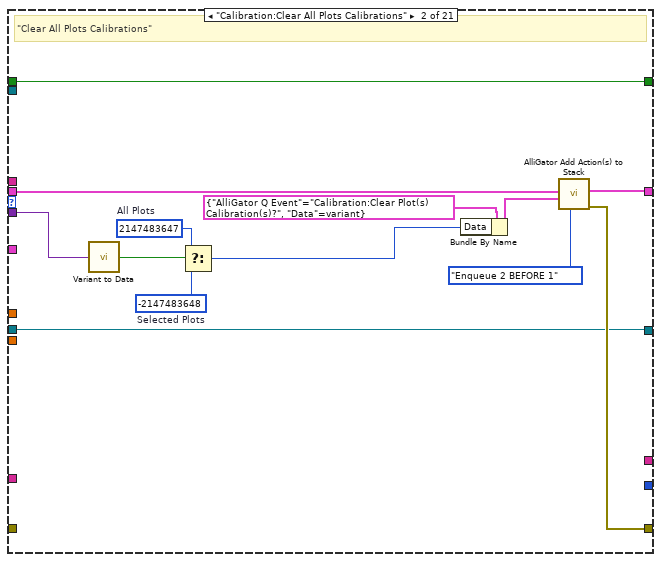
[diagram p3: hidden frame]
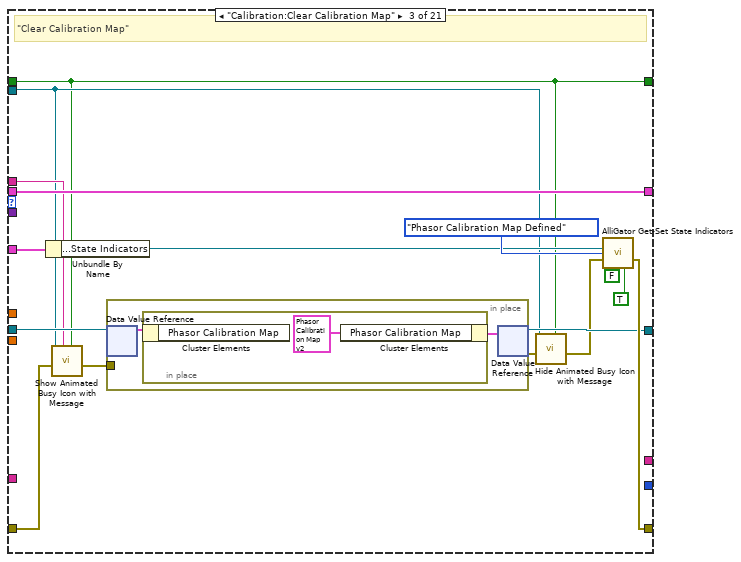
[diagram p4: hidden frame]
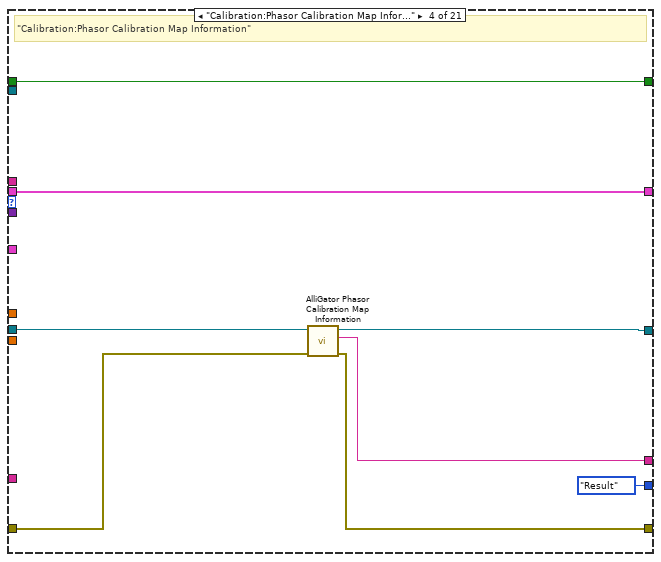
[diagram p5: hidden frame]
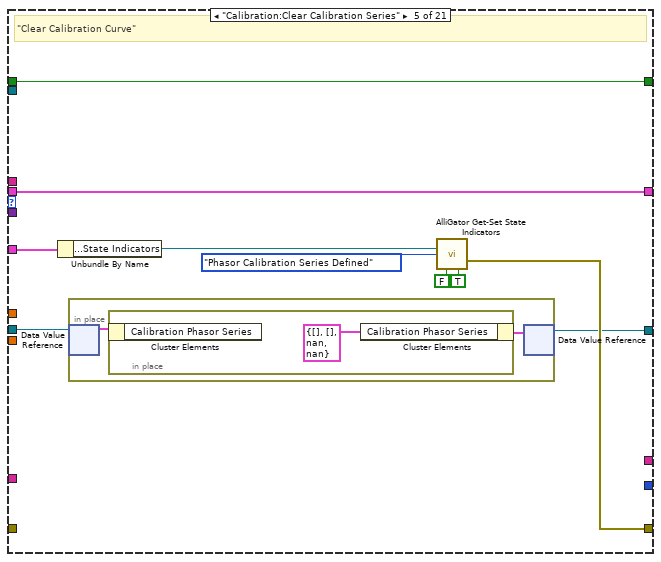
[diagram p6: hidden frame]
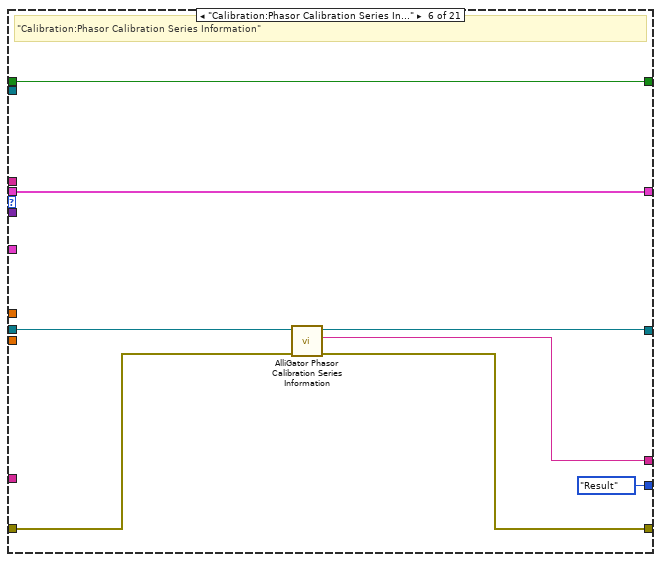
[diagram p7: hidden frame]
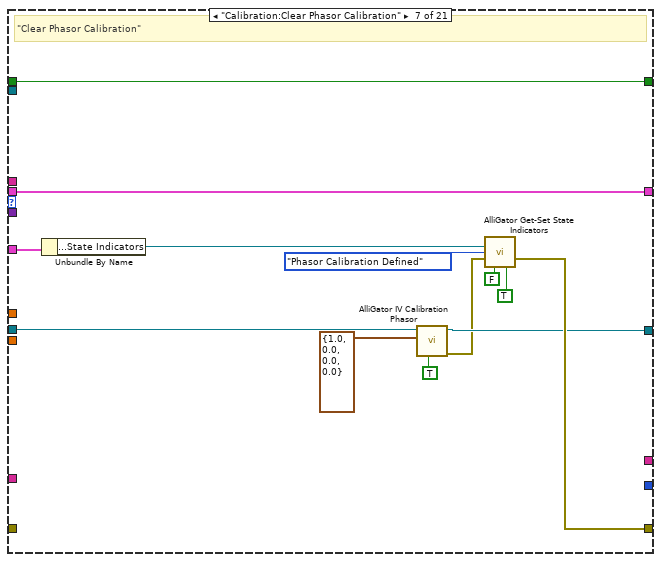
[diagram p8: hidden frame]
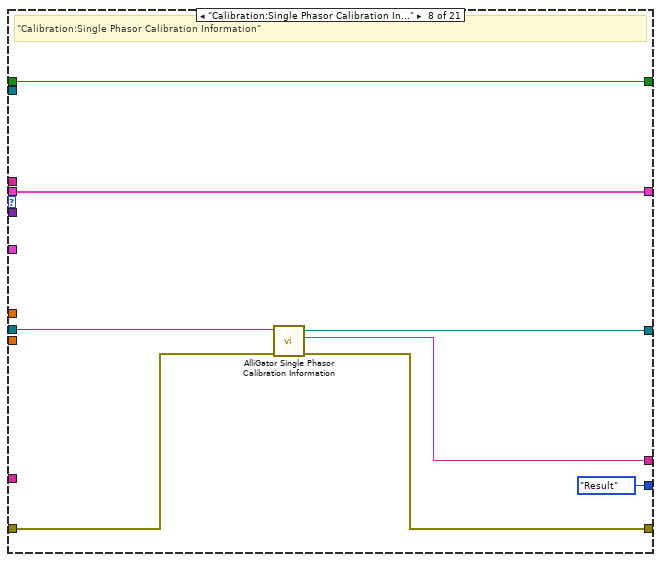
[diagram p9: hidden frame]
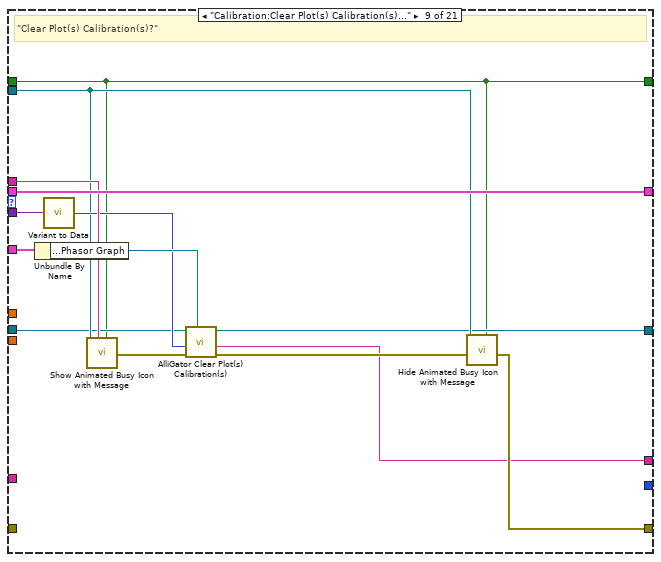
[diagram p10: hidden frame]
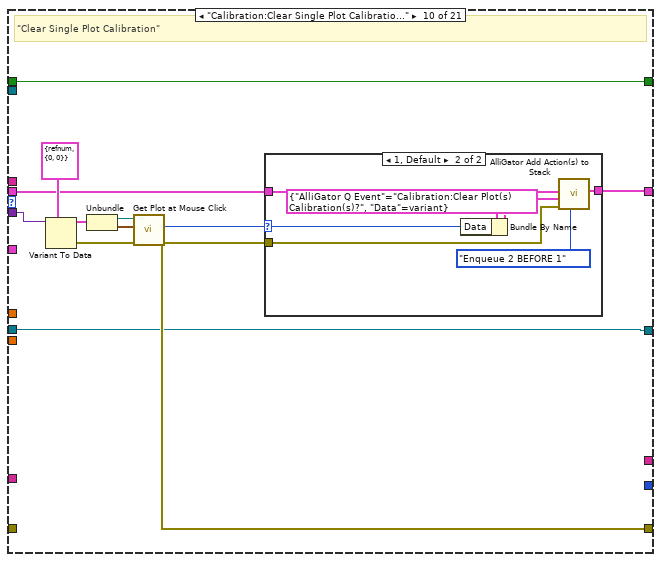
[diagram p11: hidden frame]
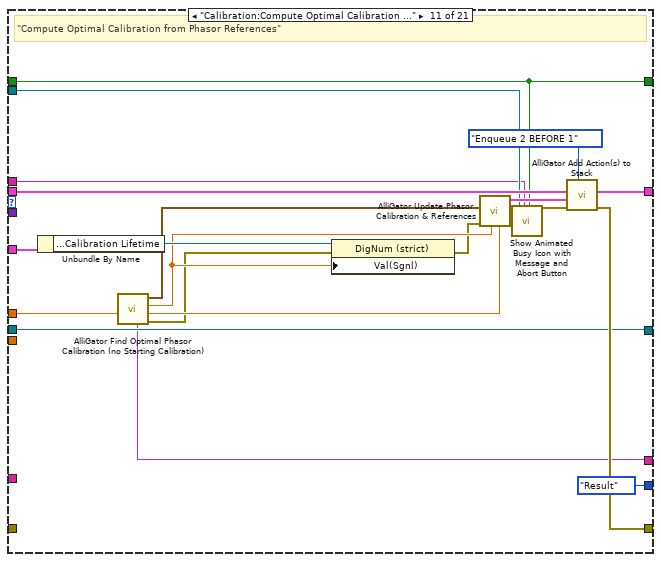
[diagram p13: hidden frame]
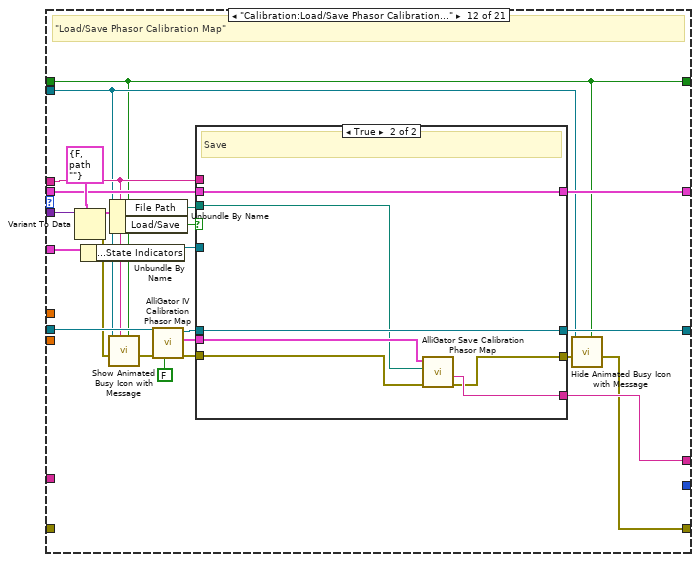
[diagram p14: hidden frame]
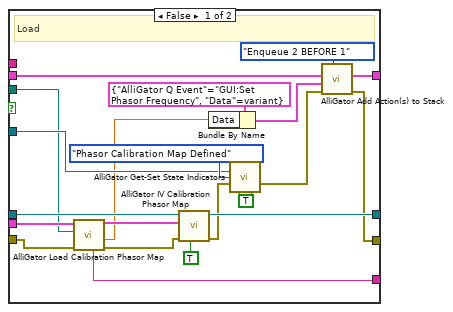
[diagram p15: hidden frame]
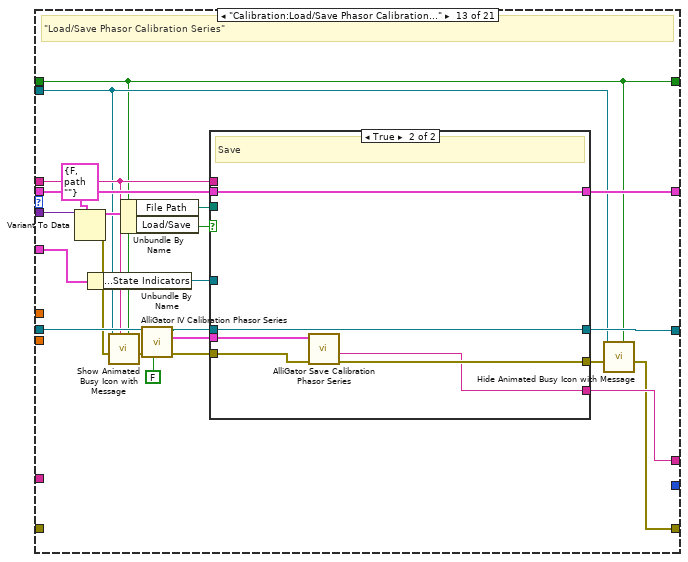
[diagram p16: hidden frame]
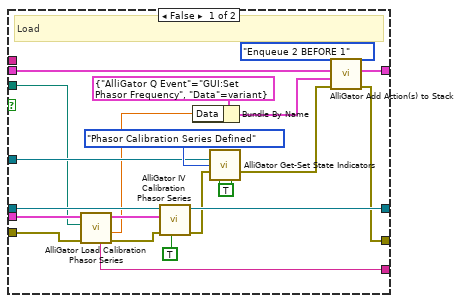
[diagram p17: hidden frame]
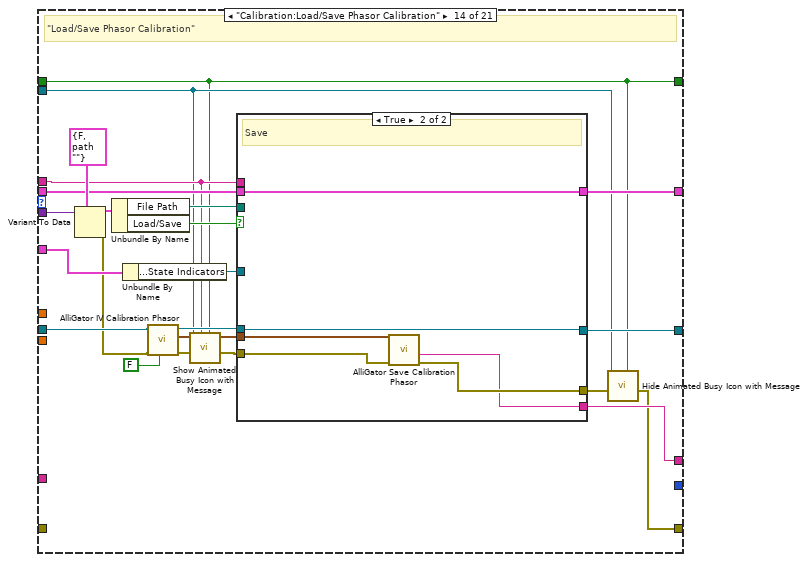
[diagram p18: hidden frame]
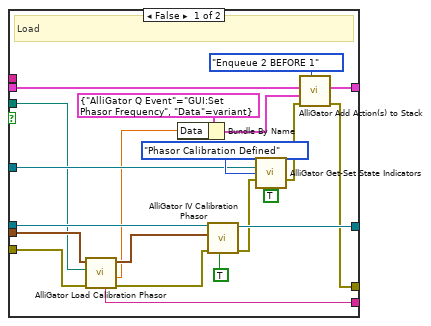
[diagram p19: hidden frame]
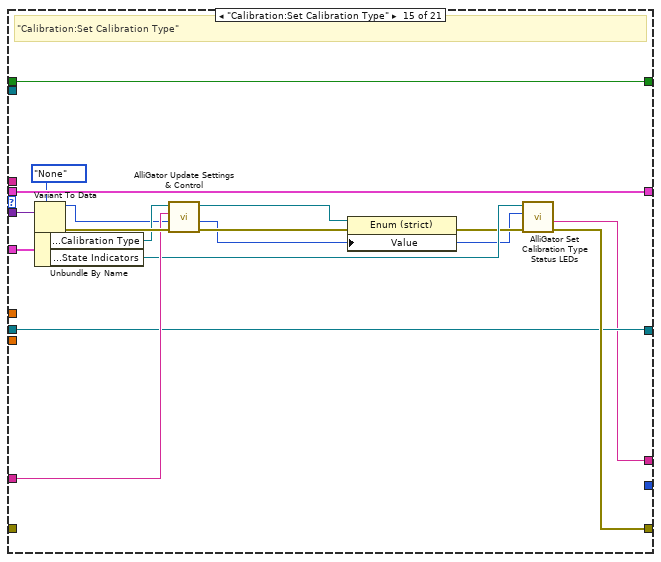
[diagram p20: hidden frame]
diagram:
  # "Author: Xavier Michalet\nCopyright 2025 REGENTS OF THE UNIVERSITY OF CALIFORNIA\n\nRedistribution and use in source and binary forms, with or without modification, are permitted provided that the following conditions are met:\n\n1. Redistributions of source code must retain the above copyright notice, this list of conditions and the following disclaimer.\n\n2. Redistributions in binary form must reproduce the above copyright notice, this list of conditions and the following disclaimer in the documentation and/or other materials provided with the distribution.\n\n3. Neither the name of the copyright holder nor the names of its contributors may be used to endorse or promote products derived from this software without specific prior written permission.\n\nTHIS SOFTWARE IS PROVIDED BY THE COPYRIGHT HOLDERS AND CONTRIBUTORS “AS IS” AND ANY EXPRESS OR IMPLIED WARRANTIES, INCLUDING, BUT NOT LIMITED TO, THE IMPLIED WARRANTIES OF MERCHANTABILITY AND FITNESS FOR A PARTICULAR PURPOSE ARE DISCLAIMED. IN NO EVENT SHALL THE COPYRIGHT HOLDER OR CONTRIBUTORS BE LIABLE FOR ANY DIRECT, INDIRECT, INCIDENTAL, SPECIAL, EXEMPLARY, OR CONSEQUENTIAL DAMAGES (INCLUDING, BUT NOT LIMITED TO, PROCUREMENT OF SUBSTITUTE GOODS OR SERVICES; LOSS OF USE, DATA, OR PROFITS; OR BUSINESS INTERRUPTION) HOWEVER CAUSED AND ON ANY THEORY OF LIABILITY, WHETHER IN CONTRACT, STRICT LIABILITY, OR TORT (INCLUDING NEGLIGENCE OR OTHERWISE) ARISING IN ANY WAY OUT OF THE USE OF THIS SOFTWARE, EVEN IF ADVISED OF THE POSSIBILITY OF SUCH DAMAGE."
  n1 = call "AlliGator Event to String.vi"("AlliGator Q Event"="AlliGator Q Event in") -> ("String"=w9:string)  [unwired: 8 in]
  n2 = call "AlliGator Calibration Lifetime.vi"() -> ("Calibration Lifetime"=w19:dbl[unit])
  n3 = call "AlliGator Phasor Frequency.vi"() -> ("Phasor Frequency"=w15:dbl[unit])
  n4 = case shown="\"Calibration:Use as Calibration\"" "AlliGator Q Event in" {
    selector: "AlliGator Q Event in" -> [_ _ _ _ _ _ _ _ _ _ _ _ _ _ _ _ _ _ w446 _ _]
    tunnel: "Data" -> [w33 w44 _ _ _ _ _ _ w132 w148 _ w197 w248 w299 w341 w350 w368 w398 w445 w485 _]
    tunnel: "AlliGator Q Elements" -> [w40 w53 w69 w80 w90 w101 w114 w122 w136 w142 w174 w184 w235 w285 w343 w356 w362 w399 w447 w486 w490]
    tunnel: [w40 w52 w69 w80 w90 w101 w114 w122 w136 w141 w172 w183 w234 w284 w343 w355 w361 w399 w447 w486 w490] -> w12
    tunnel: "VI in" -> [w30 _ w56 _ _ _ _ _ w129 _ w160 w179 w230 w280 _ _ _ w383 w429 _ _]
    tunnel: w15 -> [w23 _ _ _ _ _ _ _ _ _ w175 _ _ _ _ _ _ w394 w435 _ _]
    tunnel: [w24 w48 w55 w76 w87 w100 w111 w121 w123 w139 w159 w178 w229 w279 w342 w351 w359 w391 w432 w482 w489] -> w8
    tunnel: "Script in" -> [w24 w48 w55 w76 w87 w100 w111 w121 w123 w139 w159 w178 w229 w279 w342 w351 w359 w391 w432 w482 w489]
    tunnel: "AlliGator" ("Sender") -> [_ _ _ _ _ _ _ _ _ _ _ _ _ _ w337 _ _ _ _ _ _]
    tunnel: w9 -> [w35 _ w60 _ _ _ _ _ w134 _ w158 w181 w231 w282 _ _ _ w390 w433 _ _]
    tunnel: "error in (no error)" -> [_ _ w61 w74 _ w95 _ w117 _ _ _ _ _ _ _ _ _ _ _ _ w488]
    tunnel: [w34 w42 w66 w77 w86 w97 w110 w118 w133 w138 w170 w180 w232 w281 w335 w345 w358 w379 w434 w481 w488] -> w1
    tunnel: "AlliGator Ctrl Refnums" -> [w32 _ w65 _ w85 _ w109 _ w130 _ w168 w194 w244 w294 w338 _ _ w388 w431 w480 _]
    tunnel: w19 -> [_ _ _ _ _ _ _ _ _ _ _ _ _ _ _ _ _ w389 w430 _ _]
    tunnel: "data value reference" -> [w29 w41 w63 w79 w83 w98 w107 w120 w128 w137 w163 w192 w242 w292 w330 w344 w357 w382 w428 w477 w487]
    tunnel: [w27 w41 w62 w78 w82 w99 w106 w119 w126 w137 w163 w188 w243 w293 w330 w344 w357 w380 w427 w476 w487] -> w10
    tunnel: [w25 _ _ w75 _ w96 _ w116 w124 _ w162 w185 w236 w286 w329 _ _ w378 w426 w473 _] -> w6
    tunnel: [_ _ _ Text_Format_List."Result" ("Text Format") _ Text_Format_List."Result" ("Text Format") _ Text_Format_List."Result" ("Text Format") _ _ Text_Format_List."Result" ("Text Format") _ _ _ _ _ _ Text_Format_List."Result" ("Text Format") Text_Format_List."Result" ("Text Format") Text_Format_List."Result" ("Text Format") _] -> w3
    frame "Calibration:Apply Phasor Calibration" {
      # "\"Apply Phasor Calibration?\""
      n5 = call-poly "Variant to Data.vi"("Variant"=w33) -> ("Value"=w39:i32)  [unwired: 8 in]
      n6 = Unbundle By Name(w32) -> ("Registered Events Ctrl Refnums.Phasor Graph"=w38:refnum<vi>, "Phasor Graph Ctrl Refnums"=w31:T11)
      n7 = call "Show Animated Busy Icon with Message.vi"("Already active? (F)"=w24, "Message"=w35, "Target VI Refnum"=w30) -> ("Error Out"=w28:errorcluster)  [unwired: 8 in]
      n8 = call "AlliGator Apply Calibration Phasor(s) v2.vi"("Phasor Frequency"=w23, "Phasor Graph Ref"=w38, "Error In"=w28, "Plot Index (-1: last)"=w39, "Phasor Graph Ctrl Refnums"=w31, "AlliGator IV DVR"=w29) -> ("Error Out"=w36:errorcluster, "Calibrated Phasor"=w37:T29, "AlliGator IV DVR"=w27:refnum<data-value>, "Message"=w25:string)  [unwired: 1 in, 1 out]
      n9 = call "AlliGator Update Phasor Graph Information at Cursor.vi"("Valid?"=TRUE, "Error In"=w36, "Phasor"=w37, "Current Phasor Information Indicators"=w31) -> ("Error Out"=w26:errorcluster)  [unwired: 6 in, 1 out]
      n10 = call "Hide Animated Busy Icon with Message.vi"("Already active? (F)"=w24, "Error In"=w26, "Target VI reference"=w30) -> ("Error Out"=w34:errorcluster)  [unwired: 8 in]
    }
    frame "Calibration:Clear All Plots Calibrations" {
      w45 = -2147483648  # Selected Plots
      w46 = 2147483647  # All Plots
      # "\"Clear All Plots Calibrations\""
      n11 = call-poly "Variant to Data.vi"("Variant"=w44) -> ("Value"=w47:bool)  [unwired: 8 in]
      n12 = Select(t=w46, s=w47, f=w45) -> (s? t:f=w43:i32)
      n13 = Bundle By Name(cluster=T6 {"AlliGator Q Event"=enum."Calibration:Clear Plot(s) Calibration(s)?", "Data"=variant} ("Alligator Atomic Action"), "Data"=w43) -> (w50:T6)
      n14 = call-poly "AlliGator Add Action(s) to Stack.vi"("Elements Order in Action Stack (Default: 2 BEFORE 1)"=Alligator_Elements_Order_in_Action_Stack."Enqueue 2 BEFORE 1", "Alligator Atomic Action"=w50, "Alligator Queue Element 1"=w53) -> ("Error Out"=w42:errorcluster, "Alligator Queue Element 1 (+ 2)"=w52:T6[])  [unwired: 7 in]
    }
    frame "Calibration:Clear Calibration Map" {
      # "\"Clear Calibration Map\""
      n15 = Unbundle By Name(w65) -> ("Other AlliGator Ctrl Refnums.State Indicators"=w64:refnum<vi>)
      n16 = call "Show Animated Busy Icon with Message.vi"("Already active? (F)"=w55, "Message"=w60, "Error In"=w61, "Target VI Refnum"=w56) -> ("Error Out"=w59:errorcluster)  [unwired: 7 in]
      n17 = in-place {
        in-place-border: w59 -> [_]
        n18 = in-place-dvr #1(w63) -> (w71:T30)  [unwired: 1 out]
        n19 = in-place {
          n20 = in-place-cluster #2(w71) -> ()  [unwired: 1 out]
          n21 = in-place-cluster #2("Phasor Calibration Map"=T19 {"Phasor Frequency"=80000000.0, "Calibration Lifetime"=1e-09, "ROI Centers"=[], "ROI Descriptors"=[], "Map Resolution X"=0, "Map Resolution Y"=0, "z Array"=[]}) -> (w70:T30)
        }
        n22 = in-place-dvr #1(w70) -> (w62:refnum<data-value>, w58:errorcluster)
      }
      n23 = call "Hide Animated Busy Icon with Message.vi"("Already active? (F)"=w55, "Error In"=w58, "Target VI reference"=w56) -> ("Error Out"=w57:errorcluster)  [unwired: 8 in]
      n24 = call "AlliGator Get-Set State Indicators.vi"("State Indicators Refnum"=w64, "AlliGator State Indicators List"=AlliGator_State_Indicators_List."Phasor Calibration Map Defined" ("Time-Gated Phasor Analysis Task List"), "Error In"=w57, "ON/OFF"=FALSE ("Set (T)/Unset (F)"), "Set (T)/Get"=TRUE) -> ("Error Out"=w66:errorcluster)  [unwired: 8 in, 2 out]
    }
    frame "Calibration:Phasor Calibration Map Information" {
      # "\"Calibration:Phasor Calibration Map Information\""
      n25 = call "AlliGator Phasor Calibration Map Information.vi"("error in"=w74, "AlliGator IVDR"=w79) -> ("error out"=w77:errorcluster, "Message"=w75:string, "AlliGator IVDR"=w78:refnum<data-value>)  [unwired: 7 in]
    }
    frame "Calibration:Clear Calibration Series" {
      # "\"Clear Calibration Curve\""
      n26 = Unbundle By Name(w85) -> ("Other AlliGator Ctrl Refnums.State Indicators"=w84:refnum<vi>)
      n27 = in-place {
        n28 = in-place-dvr #3(w83) -> (w92:T30)  [unwired: 1 out]
        n29 = in-place {
          n30 = in-place-cluster #4(w92) -> ()  [unwired: 1 out]
          n31 = in-place-cluster #4("Calibration Phasor Series"=T22 {"m Array"=[], "phi Array"=[], "Phasor Frequency"=nan, "Calibration Lifetime"=nan} ("Phasor Reference Plot")) -> (w91:T30)
        }
        n32 = in-place-dvr #3(w91) -> (w82:refnum<data-value>)  [unwired: 1 out]
      }
      n33 = call "AlliGator Get-Set State Indicators.vi"("State Indicators Refnum"=w84, "AlliGator State Indicators List"=AlliGator_State_Indicators_List."Phasor Calibration Series Defined" ("Time-Gated Phasor Analysis Task List"), "ON/OFF"=FALSE ("Set (T)/Unset (F)"), "Set (T)/Get"=TRUE) -> ("Error Out"=w86:errorcluster)  [unwired: 9 in, 2 out]
    }
    frame "Calibration:Phasor Calibration Series Information" {
      # "\"Calibration:Phasor Calibration Series Information\""
      n34 = call "AlliGator Phasor Calibration Series Information.vi"("error in"=w95, "AlliGator IVDR"=w98) -> ("error out"=w97:errorcluster, "Message"=w96:string, "AlliGator IVDR"=w99:refnum<data-value>)  [unwired: 7 in]
    }
    frame "Calibration:Clear Phasor Calibration" {
      # "\"Clear Phasor Calibration\""
      n35 = Unbundle By Name(w109) -> ("Other AlliGator Ctrl Refnums.State Indicators"=w108:refnum<vi>)
      n36 = call "AlliGator IV Calibration Phasor.vi"("Get (F)/ Set (T)"=TRUE, "Calibration Phasor"=T23 {"m"=1.0, "phi"=0.0, "Phasor Frequency"=0.0, "Reference Lifetime"=0.0}, "AlliGator IV DVR in"=w107) -> ("error out"=w103:errorcluster, "AlliGator IV DVR out"=w106:refnum<data-value>)  [unwired: 6 in, 1 out]
      n37 = call "AlliGator Get-Set State Indicators.vi"("State Indicators Refnum"=w108, "AlliGator State Indicators List"=AlliGator_State_Indicators_List."Phasor Calibration Defined" ("Time-Gated Phasor Analysis Task List"), "Error In"=w103, "ON/OFF"=FALSE ("Set (T)/Unset (F)"), "Set (T)/Get"=TRUE) -> ("Error Out"=w110:errorcluster)  [unwired: 8 in, 2 out]
    }
    frame "Calibration:Single Phasor Calibration Information" {
      # "\"Calibration:Single Phasor Calibration Information\""
      n38 = call "AlliGator Single Phasor Calibration Information.vi"("error in"=w117, "AlliGator IVDR"=w120) -> ("error out"=w118:errorcluster, "Message"=w116:string, "AlliGator IVDR"=w119:refnum<data-value>)  [unwired: 7 in]
    }
    frame "Calibration:Clear Plot(s) Calibration(s)?" {
      # "\"Clear Plot(s) Calibration(s)?\""
      n39 = Unbundle By Name(w130) -> ("Registered Events Ctrl Refnums.Phasor Graph"=w135:refnum<vi>)
      n40 = call-poly "Variant to Data.vi"("Variant"=w132) -> ("Value"=w131:i32)  [unwired: 8 in]
      n41 = call "Show Animated Busy Icon with Message.vi"("Already active? (F)"=w123, "Message"=w134, "Target VI Refnum"=w129) -> ("Error Out"=w127:errorcluster)  [unwired: 8 in]
      n42 = call "AlliGator Clear Plot(s) Calibration(s).vi"("Phasor Graph Ref"=w135, "Error In"=w127, "Plot Index (-1: last)"=w131, "AlliGator IV DVR"=w128) -> ("Error Out"=w125:errorcluster, "Message"=w124:string, "AlliGator IV DVR"=w126:refnum<data-value>)  [unwired: 4 in, 1 out]
      n43 = call "Hide Animated Busy Icon with Message.vi"("Already active? (F)"=w123, "Error In"=w125, "Target VI reference"=w129) -> ("Error Out"=w133:errorcluster)  [unwired: 8 in]
    }
    frame "Calibration:Clear Single Plot Calibration" {
      # "\"Clear Single Plot Calibration\""
      n44 = Variant To Data(type=T24 {"Multiplot XY Graph"=refnum, "Mouse Coordinates"={"Horizontal"=0, "Vertical"=0}} ("Mouse Click Event Data"), Variant=w148) -> (data=w146:T24, error out=w143:errorcluster)  [unwired: 1 in]
      n45 = Unbundle(w146) -> ("Multiplot XY Graph"=w145:T25, "Mouse Coordinates"=w144:T26)
      n46 = call-poly "Get Plot at Mouse Click.vi"("error in (no error)"=w143, "Mouse Click Coordinates"=w144, "XY Graph in"=w145) -> ("error out"=w138:errorcluster, "Plot at Coordinates"=w140:i32)  [unwired: 2 in, 5 out]
      n47 = case shown="1, Default" w140 {
        selector: w140 -> [_ w150]
        tunnel: w142 -> [w149 w156]
        tunnel: [w149 w155] -> w141
        tunnel: w138 -> [_ w154]
        frame 0 {
          # "The first plot is the UC"
        }
        frame 1, Default {
          n48 = Bundle By Name(cluster=T6 {"AlliGator Q Event"=enum."Calibration:Clear Plot(s) Calibration(s)?", "Data"=variant} ("Alligator Atomic Action"), "Data"=w150) -> (w152:T6)
          n49 = call-poly "AlliGator Add Action(s) to Stack.vi"("Elements Order in Action Stack (Default: 2 BEFORE 1)"=Alligator_Elements_Order_in_Action_Stack."Enqueue 2 BEFORE 1", "Error In"=w154, "Alligator Atomic Action"=w152, "Alligator Queue Element 1"=w156) -> ("Alligator Queue Element 1 (+ 2)"=w155:T6[])  [unwired: 6 in, 1 out]
        }
      }
    }
    frame "Calibration:Compute Optimal Calibration from Phasor References" {
      # "\"Compute Optimal Calibration from Phasor References\""
      n50 = Unbundle By Name(w168) -> ("Phasor Graph Ctrl Refnums.Calibration Lifetime"=w167:refnum<vi>)
      n51 = call "AlliGator Find Optimal Phasor Calibration (no Starting Calibration).vi"("Phasor Frequency"=w175) -> ("Error Out"=w165:errorcluster, "tau 2"=w176:dbl[unit], "tau 1"=w166:dbl[unit], "Calibration Phasor (g, s)"=w177:T29, "Message"=w162:string)  [unwired: 6 in]
      n52 = property class="DigNum (strict)"(reference=w167, error in=w165, "Val(Sgnl)"=w166) -> (error out=w164:errorcluster)  [unwired: 1 out]
      n53 = call "AlliGator Update Phasor Calibration & References.vi"("tau 2"=w176, "tau 1"=w166, "error in (no error)"=w164, "Calibration Phasor"=w177) -> ("Error Out"=w171:errorcluster, "Named Q Element out"=w173:T6[])  [unwired: 6 in]
      n54 = call "Show Animated Busy Icon with Message and Abort Button.vi"("Already active? (F)"=w159, "Message"=w158, "Target VI reference"=w160, "Error In"=w171) -> ("Error Out"=w161:errorcluster)  [unwired: 15 in]
      n55 = call-poly "AlliGator Add Action(s) to Stack.vi"("Elements Order in Action Stack (Default: 2 BEFORE 1)"=Alligator_Elements_Order_in_Action_Stack."Enqueue 2 BEFORE 1", "Error In"=w161, "Alligator Queue Element 2"=w173, "Alligator Queue Element 1"=w174) -> ("Error Out"=w170:errorcluster, "Alligator Queue Element 1 (+ 2)"=w172:T6[])  [unwired: 6 in]
    }
    frame "Calibration:Load/Save Phasor Calibration Map" {
      # "\"Load/Save Phasor Calibration Map\""
      n56 = Variant To Data(type=T27 {"Load/Save"=FALSE, "File Path"=path ""}, Variant=w197) -> (data=w199:T27, error out=w191:errorcluster)  [unwired: 1 in]
      n57 = Unbundle By Name(w194) -> ("Other AlliGator Ctrl Refnums.State Indicators"=w193:refnum<vi>)
      n58 = call "Show Animated Busy Icon with Message.vi"("Already active? (F)"=w178, "Message"=w181, "Error In"=w191, "Target VI Refnum"=w179) -> ("Error Out"=w182:errorcluster)  [unwired: 7 in]
      n59 = Unbundle By Name(w199) -> ("File Path"=w195:path, "Load/Save"=w196:bool)
      n60 = call "AlliGator IV Calibration Phasor Map.vi"("Get (F)/ Set (T)"=FALSE, "error in (no error)"=w182, "AlliGator IV DVR in"=w192) -> ("error out"=w187:errorcluster, "Phasor Calibration Map"=w190:T19, "AlliGator IV DVR out"=w189:refnum<data-value>)  [unwired: 6 in]
      n61 = case shown="True" w196 {
        tunnel: w193 -> [w220 _]
        tunnel: [w206 w223] -> w200
        tunnel: w181 -> [_ _]
        tunnel: w195 -> [w214 w226]
        tunnel: w190 -> [w219 w228]
        tunnel: w189 -> [w218 w227]
        tunnel: [w217 w227] -> w188
        tunnel: w187 -> [w202 w224]
        tunnel: [w205 w225] -> w185
        tunnel: w184 -> [w209 w222]
        tunnel: [w208 w222] -> w183
        frame False {
          w203 = TRUE ("Set (T)/Unset (F)")
          # "Load"
          n62 = call "AlliGator Load Calibration Phasor Map.vi"("Error In"=w202, "File Path (empty: dialog)"=w214, "Calibration Phasor Map in"=w219) -> ("error out"=w201:errorcluster, "Phasor Frequency"=w204:dbl[unit], "Calibration Phasor Map out"=w216:T19, "Message"=w205:string)  [unwired: 4 in, 1 out]
          n63 = call "AlliGator IV Calibration Phasor Map.vi"("Get (F)/ Set (T)"=TRUE, "error in (no error)"=w201, "Phasor Calibration Map 2"=w216, "AlliGator IV DVR in"=w218) -> ("error out"=w213:errorcluster, "AlliGator IV DVR out"=w217:refnum<data-value>)  [unwired: 5 in, 1 out]
          n64 = Bundle By Name(cluster=T6 {"AlliGator Q Event"=enum."GUI:Set Phasor Frequency", "Data"=variant} ("Alligator Atomic Action"), "Data"=w204) -> (w210:T6)
          n65 = call "AlliGator Get-Set State Indicators.vi"("State Indicators Refnum"=w220, "AlliGator State Indicators List"=AlliGator_State_Indicators_List."Phasor Calibration Map Defined" ("Time-Gated Phasor Analysis Task List"), "Error In"=w213, "ON/OFF"=w203, "Set (T)/Get"=w203) -> ("Error Out"=w207:errorcluster)  [unwired: 8 in, 2 out]
          n66 = call-poly "AlliGator Add Action(s) to Stack.vi"("Elements Order in Action Stack (Default: 2 BEFORE 1)"=Alligator_Elements_Order_in_Action_Stack."Enqueue 2 BEFORE 1", "Error In"=w207, "Alligator Atomic Action"=w210, "Alligator Queue Element 1"=w209) -> ("Error Out"=w206:errorcluster, "Alligator Queue Element 1 (+ 2)"=w208:T6[])  [unwired: 6 in]
        }
        frame True {
          # "Save"
          n67 = call "AlliGator Save Calibration Phasor Map.vi"("Error In"=w224, "File Path (empty: dialog)"=w226, "Calibration Phasor Map"=w228) -> ("error out"=w223:errorcluster, "Message"=w225:string)  [unwired: 6 in, 1 out]
        }
      }
      n68 = call "Hide Animated Busy Icon with Message.vi"("Already active? (F)"=w178, "Error In"=w200, "Target VI reference"=w179) -> ("Error Out"=w180:errorcluster)  [unwired: 8 in]
    }
    frame "Calibration:Load/Save Phasor Calibration Series" {
      # "\"Load/Save Phasor Calibration Series\""
      n69 = Variant To Data(type=T27 {"Load/Save"=FALSE, "File Path"=path ""}, Variant=w248) -> (data=w249:T27, error out=w241:errorcluster)  [unwired: 1 in]
      n70 = Unbundle By Name(w244) -> ("Other AlliGator Ctrl Refnums.State Indicators"=w250:refnum<vi>)
      n71 = call "Show Animated Busy Icon with Message.vi"("Already active? (F)"=w229, "Message"=w231, "Error In"=w241, "Target VI Refnum"=w230) -> ("Error Out"=w233:errorcluster)  [unwired: 7 in]
      n72 = Unbundle By Name(w249) -> ("File Path"=w245:path, "Load/Save"=w246:bool)
      n73 = call "AlliGator IV Calibration Phasor Series.vi"("Get (F)/ Set (T)"=FALSE, "error in (no error)"=w233, "AlliGator IV DVR in"=w242) -> ("error out"=w239:errorcluster, "Calibration Phasor Series"=w237:T22, "AlliGator IV DVR out"=w240:refnum<data-value>)  [unwired: 6 in]
      n74 = case shown="True" w246 {
        tunnel: [w257 w278] -> w251
        tunnel: w250 -> [w271 _]
        tunnel: w231 -> [_ _]
        tunnel: w245 -> [w265 _]
        tunnel: w239 -> [w253 w273]
        tunnel: w240 -> [w270 w277]
        tunnel: [w269 w277] -> w243
        tunnel: w237 -> [w266 w276]
        tunnel: [w255 w275] -> w236
        tunnel: w235 -> [w260 w274]
        tunnel: [w259 w274] -> w234
        frame False {
          w254 = TRUE ("Set (T)/Unset (F)")
          # "Load"
          n75 = call "AlliGator Load Calibration Phasor Series.vi"("Error In"=w253, "File Path"=w265, "Calibration Phasor Series in"=w266) -> ("error out"=w252:errorcluster, "Phasor Frequency"=w256:dbl[unit], "Calibration Phasor Series out"=w268:T22, "Message"=w255:string)  [unwired: 4 in, 1 out]
          n76 = call "AlliGator IV Calibration Phasor Series.vi"("Get (F)/ Set (T)"=TRUE, "error in (no error)"=w252, "Calibration Phasor Series"=w268, "AlliGator IV DVR in"=w270) -> ("error out"=w264:errorcluster, "AlliGator IV DVR out"=w269:refnum<data-value>)  [unwired: 5 in, 1 out]
          n77 = Bundle By Name(cluster=T6 {"AlliGator Q Event"=enum."GUI:Set Phasor Frequency", "Data"=variant} ("Alligator Atomic Action"), "Data"=w256) -> (w261:T6)
          n78 = call "AlliGator Get-Set State Indicators.vi"("State Indicators Refnum"=w271, "AlliGator State Indicators List"=AlliGator_State_Indicators_List."Phasor Calibration Series Defined" ("Time-Gated Phasor Analysis Task List"), "Error In"=w264, "ON/OFF"=w254, "Set (T)/Get"=w254) -> ("Error Out"=w258:errorcluster)  [unwired: 8 in, 2 out]
          n79 = call-poly "AlliGator Add Action(s) to Stack.vi"("Elements Order in Action Stack (Default: 2 BEFORE 1)"=Alligator_Elements_Order_in_Action_Stack."Enqueue 2 BEFORE 1", "Error In"=w258, "Alligator Atomic Action"=w261, "Alligator Queue Element 1"=w260) -> ("Error Out"=w257:errorcluster, "Alligator Queue Element 1 (+ 2)"=w259:T6[])  [unwired: 6 in]
        }
        frame True {
          # "Save"
          n80 = call "AlliGator Save Calibration Phasor Series.vi"("Error In"=w273, "Calibration Phasor Series"=w276) -> ("error out"=w278:errorcluster, "Message"=w275:string)  [unwired: 7 in, 1 out]
        }
      }
      n81 = call "Hide Animated Busy Icon with Message.vi"("Already active? (F)"=w229, "Error In"=w251, "Target VI reference"=w230) -> ("Error Out"=w232:errorcluster)  [unwired: 8 in]
    }
    frame "Calibration:Load/Save Phasor Calibration" {
      # "\"Load/Save Phasor Calibration\""
      n82 = Variant To Data(type=T27 {"Load/Save"=FALSE, "File Path"=path ""}, Variant=w299) -> (data=w297:T27, error out=w291:errorcluster)  [unwired: 1 in]
      n83 = Unbundle By Name(w297) -> ("File Path"=w295:path, "Load/Save"=w296:bool)
      n84 = Unbundle By Name(w294) -> ("Other AlliGator Ctrl Refnums.State Indicators"=w300:refnum<vi>)
      n85 = call "AlliGator IV Calibration Phasor.vi"("Get (F)/ Set (T)"=FALSE, "error in (no error)"=w291, "AlliGator IV DVR in"=w292) -> ("error out"=w289:errorcluster, "Calibration Phasor"=w287:T23, "AlliGator IV DVR out"=w290:refnum<data-value>)  [unwired: 6 in]
      n86 = call "Show Animated Busy Icon with Message.vi"("Already active? (F)"=w279, "Message"=w282, "Error In"=w289, "Target VI Refnum"=w280) -> ("Error Out"=w283:errorcluster)  [unwired: 7 in]
      n87 = case shown="True" w296 {
        tunnel: w300 -> [w321 _]
        tunnel: [w303 w328] -> w301
        tunnel: w282 -> [_ _]
        tunnel: w295 -> [w313 _]
        tunnel: w283 -> [w316 w326]
        tunnel: w290 -> [w319 w327]
        tunnel: [w317 w327] -> w293
        tunnel: w287 -> [w314 w325]
        tunnel: [w312 w324] -> w286
        tunnel: w285 -> [w311 w323]
        tunnel: [w306 w323] -> w284
        frame False {
          w302 = TRUE ("Set (T)/Unset (F)")
          # "Load"
          n88 = call "AlliGator Load Calibration Phasor.vi"("Error In"=w316, "File Path"=w313, "Calibration Phasor in"=w314) -> ("error out"=w320:errorcluster, "Phasor Frequency"=w308:dbl[unit], "Calibration Phasor out"=w318:T23, "Message"=w312:string)  [unwired: 4 in, 1 out]
          n89 = Bundle By Name(cluster=T6 {"AlliGator Q Event"=enum."GUI:Set Phasor Frequency", "Data"=variant} ("Alligator Atomic Action"), "Data"=w308) -> (w307:T6)
          n90 = call "AlliGator IV Calibration Phasor.vi"("Get (F)/ Set (T)"=TRUE, "error in (no error)"=w320, "Calibration Phasor"=w318, "AlliGator IV DVR in"=w319) -> ("error out"=w305:errorcluster, "AlliGator IV DVR out"=w317:refnum<data-value>)  [unwired: 5 in, 1 out]
          n91 = call "AlliGator Get-Set State Indicators.vi"("State Indicators Refnum"=w321, "AlliGator State Indicators List"=AlliGator_State_Indicators_List."Phasor Calibration Defined" ("Time-Gated Phasor Analysis Task List"), "Error In"=w305, "ON/OFF"=w302, "Set (T)/Get"=w302) -> ("Error Out"=w304:errorcluster)  [unwired: 8 in, 2 out]
          n92 = call-poly "AlliGator Add Action(s) to Stack.vi"("Elements Order in Action Stack (Default: 2 BEFORE 1)"=Alligator_Elements_Order_in_Action_Stack."Enqueue 2 BEFORE 1", "Error In"=w304, "Alligator Atomic Action"=w307, "Alligator Queue Element 1"=w311) -> ("Error Out"=w303:errorcluster, "Alligator Queue Element 1 (+ 2)"=w306:T6[])  [unwired: 6 in]
        }
        frame True {
          # "Save"
          n93 = call "AlliGator Save Calibration Phasor.vi"("Error In"=w326, "Calibration Phasor"=w325) -> ("error out"=w328:errorcluster, "Message"=w324:string)  [unwired: 7 in, 1 out]
        }
      }
      n94 = call "Hide Animated Busy Icon with Message.vi"("Already active? (F)"=w279, "Error In"=w301, "Target VI reference"=w280) -> ("Error Out"=w281:errorcluster)  [unwired: 8 in]
    }
    frame "Calibration:Set Calibration Type" {
      # "\"Calibration:Set Calibration Type\""
      n95 = Variant To Data(type=Phasor_Calibration_Type."None" ("Calibration Type"), Variant=w341) -> (data=w331:T28, error out=w339:errorcluster)  [unwired: 1 in]
      n96 = Unbundle By Name(w338) -> ("Phasor Graph Ctrl Refnums.Calibration Type"=w332:refnum<vi>, "Other AlliGator Ctrl Refnums.State Indicators"=w336:refnum<vi>)
      n97 = call "AlliGator Update Settings & Control.vi"("Error In"=w339, "Value"=w331, "Sender"=w337, "CtlRef"=w332) -> ("Error Out"=w334:errorcluster)  [unwired: 7 in]
      n98 = property class="Enum (strict)"(reference=w332, error in=w334, "Value"=w331) -> (error out=w333:errorcluster)  [unwired: 1 out]
      n99 = call "AlliGator Set Calibration Type Status LEDs.vi"("error in (no error)"=w333, "Calibration Type"=w331, "State Indicators"=w336) -> ("error out"=w335:errorcluster, "Message"=w329:string)  [unwired: 7 in]
    }
    frame "Calibration:Update Multiple Plots Calibration" {
      w346 = -2147483648  # Selected Plots: -2^31
      w348 = 2147483647  # All Plots: 2^31-1
      # "\"Update All Plots Calibrations\""
      n100 = call-poly "Variant to Data.vi"("Variant"=w350) -> ("Value"=w349:bool)  [unwired: 8 in]
      n101 = Select(t=w348, s=w349, f=w346) -> (s? t:f=w347:i32)
      n102 = Bundle By Name(cluster=T6 {"AlliGator Q Event"=enum."Calibration:Apply Phasor Calibration", "Data"=variant} ("Alligator Atomic Action"), "Data"=w347) -> (w353:T6)
      n103 = call-poly "AlliGator Add Action(s) to Stack.vi"("Elements Order in Action Stack (Default: 2 BEFORE 1)"=Alligator_Elements_Order_in_Action_Stack."Enqueue 2 BEFORE 1", "Alligator Atomic Action"=w353, "Alligator Queue Element 1"=w356) -> ("Error Out"=w345:errorcluster, "Alligator Queue Element 1 (+ 2)"=w355:T6[])  [unwired: 7 in]
    }
    frame "Calibration:Update Single Plot Calibration" {
      # "\"Update Single Plot Calibration\""
      n104 = Variant To Data(type=T24 {"Multiplot XY Graph"=refnum, "Mouse Coordinates"={"Horizontal"=0, "Vertical"=0}} ("Mouse Click Event Data"), Variant=w368) -> (data=w366:T24, error out=w363:errorcluster)  [unwired: 1 in]
      n105 = Unbundle(w366) -> ("Multiplot XY Graph"=w365:T25, "Mouse Coordinates"=w364:T26)
      n106 = call-poly "Get Plot at Mouse Click.vi"("error in (no error)"=w363, "Mouse Click Coordinates"=w364, "XY Graph in"=w365) -> ("error out"=w358:errorcluster, "Plot at Coordinates"=w360:i32)  [unwired: 2 in, 5 out]
      n107 = case shown="1, Default" w360 {
        selector: w360 -> [_ w370]
        tunnel: w362 -> [w369 w376]
        tunnel: [w369 w375] -> w361
        tunnel: w358 -> [_ w374]
        frame 0 {
          # "The first plot is the UC"
        }
        frame 1, Default {
          n108 = Bundle By Name(cluster=T6 {"AlliGator Q Event"=enum."Calibration:Apply Phasor Calibration", "Data"=variant} ("Alligator Atomic Action"), "Data"=w370) -> (w372:T6)
          n109 = call-poly "AlliGator Add Action(s) to Stack.vi"("Elements Order in Action Stack (Default: 2 BEFORE 1)"=Alligator_Elements_Order_in_Action_Stack."Enqueue 2 BEFORE 1", "Error In"=w374, "Alligator Atomic Action"=w372, "Alligator Queue Element 1"=w376) -> ("Alligator Queue Element 1 (+ 2)"=w375:T6[])  [unwired: 6 in, 1 out]
        }
      }
    }
    frame "Calibration:Use as Calibration Map" {
      # "\"Use as Calibration Map\""
      n110 = Unbundle By Name(w388) -> ("Other AlliGator Ctrl Refnums.State Indicators"=w392:refnum<vi>)
      n111 = Variant To Data(type=T24 {"Multiplot XY Graph"=refnum, "Mouse Coordinates"={"Horizontal"=0, "Vertical"=0}} ("Mouse Click Event Data"), Variant=w398) -> (data=w386:T24, error out=w393:errorcluster)  [unwired: 1 in]
      n112 = Unbundle(w386) -> ("Multiplot XY Graph"=w385:T25, "Mouse Coordinates"=w384:T26)
      n113 = call-poly "Get Plot at Mouse Click.vi"("error in (no error)"=w393, "Mouse Click Coordinates"=w384, "XY Graph in"=w385) -> ("error out"=w381:errorcluster, "Plot at Coordinates"=w396:i32, "XY Graph out"=w397:T25, "Plot Name"=w395:string)  [unwired: 2 in, 3 out]
      n114 = case shown="1, Default" w396 {
        selector: w396 -> [_ w410]
        tunnel: w394 -> [_ w418]
        tunnel: w397 -> [_ _]
        tunnel: w389 -> [_ w417]
        tunnel: w395 -> [_ w415]
        tunnel: w381 -> [w400 w416]
        tunnel: w392 -> [_ w413]
        tunnel: w391 -> [_ w404]
        tunnel: w390 -> [_ w411]
        tunnel: w383 -> [_ w409]
        tunnel: w382 -> [w401 w408]
        tunnel: [w401 w407] -> w380
        tunnel: [w400 w406] -> w379
        tunnel: [_ w405] -> w378
        frame 0 {
          # "UC or SEPL"
        }
        frame 1, Default {
          n115 = call "Show Animated Busy Icon with Message.vi"("Already active? (F)"=w404, "Message"=w411, "Error In"=w416, "Target VI Refnum"=w409) -> ("Error Out"=w412:errorcluster)  [unwired: 7 in]
          n116 = call "AlliGator Use Phasor Plot as Phasor Calibration Map.vi"("Calibration Lifetime"=w417, "Phasor Frequency"=w418, "error in (no error)"=w412, "Plot Name"=w415, "Phasor Graph Plot index"=w410, "Data Value Reference in"=w408) -> ("error out"=w403:errorcluster, "Message"=w405:string, "Valid Map?"=w414:bool, "Data Value Reference out"=w407:refnum<data-value>)  [unwired: 2 in]
          n117 = case shown="True" w414 {
            tunnel: w413 -> [_ w423]
            tunnel: w403 -> [w419 w422]
            tunnel: [w419 w421] -> w402
            frame False {
              n118 = call "Play Error Sound.vi"() -> ()  [unwired: 27 in, 1 out]
            }
            frame True {
              w420 = TRUE ("Set (T)/Unset (F)")
              n119 = call "AlliGator Get-Set State Indicators.vi"("State Indicators Refnum"=w423, "AlliGator State Indicators List"=AlliGator_State_Indicators_List."Phasor Calibration Map Defined" ("Time-Gated Phasor Analysis Task List"), "Error In"=w422, "ON/OFF"=w420, "Set (T)/Get"=w420) -> ("Error Out"=w421:errorcluster)  [unwired: 8 in, 2 out]
            }
          }
          n120 = call "Hide Animated Busy Icon with Message.vi"("Already active? (F)"=w404, "Error In"=w402, "Target VI reference"=w409) -> ("Error Out"=w406:errorcluster)  [unwired: 8 in]
        }
      }
    }
    frame "Calibration:Use as Calibration Series" {
      # "\"Use as Calibration Series\""
      n121 = Variant To Data(type=T24 {"Multiplot XY Graph"=refnum, "Mouse Coordinates"={"Horizontal"=0, "Vertical"=0}} ("Mouse Click Event Data"), Variant=w445) -> (data=w443:T24, error out=w440:errorcluster)  [unwired: 1 in]
      n122 = Unbundle(w443) -> ("Multiplot XY Graph"=w442:T25, "Mouse Coordinates"=w441:T26)
      n123 = call-poly "Get Plot at Mouse Click.vi"("error in (no error)"=w440, "Mouse Click Coordinates"=w441, "XY Graph in"=w442) -> ("error out"=w439:errorcluster, "Plot at Coordinates"=w437:i32, "XY Graph out"=w438:T25, "Plot Name"=w436:string)  [unwired: 2 in, 3 out]
      n124 = case shown="1, Default" w437 {
        selector: w437 -> [_ w467]
        tunnel: w446 -> [_ w470]
        tunnel: w435 -> [_ w469]
        tunnel: w439 -> [w448 w468]
        tunnel: w438 -> [_ _]
        tunnel: w430 -> [_ w465]
        tunnel: w428 -> [w449 w464]
        tunnel: [w449 w463] -> w427
        tunnel: w436 -> [_ w462]
        tunnel: [w448 w452] -> w434
        tunnel: w433 -> [_ w458]
        tunnel: w432 -> [_ w451]
        tunnel: w431 -> [_ w456]
        tunnel: w429 -> [_ w454]
        tunnel: [_ w453] -> w426
        frame ..0 {
          # "not found (<0) or UC (0)"
        }
        frame 1, Default {
          w450 = TRUE ("Set (T)/Unset (F)")
          n125 = call "Show Animated Busy Icon with Message.vi"("Already active? (F)"=w451, "Message"=w458, "Error In"=w468, "Target VI Refnum"=w454) -> ("Error Out"=w459:errorcluster)  [unwired: 7 in]
          n126 = Unbundle By Name(w456) -> ("Other AlliGator Ctrl Refnums.State Indicators"=w455:refnum<vi>)
          n127 = call "AlliGator Use Phasor Plot as Phasor Calibration Series.vi"("Calibration Lifetime"=w465, "Phasor Frequency"=w469, "error in (no error)"=w459, "Phasor Graph Plot index"=w467, "Data Value Reference in"=w464) -> ("error out"=w460:errorcluster, "Data Value Reference out"=w463:refnum<data-value>)  [unwired: 5 in]
          n128 = call "Hide Animated Busy Icon with Message.vi"("Already active? (F)"=w451, "Error In"=w460, "Target VI reference"=w454) -> ("Error Out"=w457:errorcluster)  [unwired: 8 in]
          n129 = Format Into String(format string="%s: %s", error in=w457, w470, w462) -> (resulting string=w453:string, error out=w452:errorcluster)  [unwired: 1 in]
          n130 = call "AlliGator Get-Set State Indicators.vi"("State Indicators Refnum"=w455, "AlliGator State Indicators List"=AlliGator_State_Indicators_List."Phasor Calibration Series Defined" ("Time-Gated Phasor Analysis Task List"), "Error In"=w457, "ON/OFF"=w450, "Set (T)/Get"=w450) -> ()  [unwired: 8 in, 3 out]
        }
      }
    }
    frame "Calibration:Use as Calibration" {
      w472 = TRUE ("Set (T)/Unset (F)")
      # "\"Use as Calibration\""
      n131 = Unbundle By Name(w480) -> ("Other AlliGator Ctrl Refnums.State Indicators"=w479:refnum<vi>)
      n132 = Variant To Data(type=T29 {"g"=0.0, "s"=0.0} ("Phasor (g, s)"), Variant=w485) -> (data=w474:T29, error out=w483:errorcluster)  [unwired: 1 in]
      n133 = Unbundle By Name(w483) -> ("status"=w475:bool)
      n134 = call "AlliGator Update IV Calibration Phasor.vi"("Phasor"=w474, "Use Last Raw Phasor"=w475, "AlliGator IV DVR in"=w477) -> ("error out"=w481:errorcluster, "Message"=w473:string, "AlliGator IV DVR out"=w476:refnum<data-value>)  [unwired: 6 in]
      n135 = call "AlliGator Get-Set State Indicators.vi"("State Indicators Refnum"=w479, "AlliGator State Indicators List"=AlliGator_State_Indicators_List."Phasor Calibration Defined" ("Time-Gated Phasor Analysis Task List"), "ON/OFF"=w472, "Set (T)/Get"=w472) -> ()  [unwired: 9 in, 3 out]
    }
    frame Default {
      # "\"---- Phasor Calibration ----\""
    }
  }
  "error out" <- w1
  "Alligator Queue Element 1 (+ 2)" <- w12
  "AlliGator IV DVR" <- w10
  "Script out" <- w8
  n136 = call "Get Current Message Text Format.vi"("Text Format"=w3) -> ("Error Out"=w2:errorcluster, "Message Formatting"=w5:T2)  [unwired: 8 in]
  n137 = call "AlliGator Package Notebook Messages.vi"("Error In"=w2, "Message Formatting"=w5, "Message"=w6, "AlliGator Q Event in"="AlliGator Q Event in") -> ("[Notebook Message]"=→"[Notebook Message]":T1[])  [unwired: 6 in, 1 out]
